vi "SetROI_v4.vi"() -> ()   [LabVIEW 2015]
uses:
  <vilib>/Utility/miscctls.llb/LVPoint32TypeDef.ctl
panel:
  in  "imageselect":u16(ring)
  in  "Add":bool
  in  "Rotate":bool
  in  "Array":T1[](array[typedef])
  in  "no draw":bool
  in  "Scanning Mode":u16(ring) items=["Raster", "Spiral", "resonant"]
  in  "reset angle":bool
  out "Angle":dbl
  in  "Drawing Mode":u16(ring) items=["Image", "Fill Rectangle", "Fill Circle", "Draw Freeform", "Fill Freeform", "Ellipse ", "Line"]
  in  "square matrix":bool
  in  "square pixels":bool
  in  "Ypixels":i32
  in  "Xpixels":i32
  out "Vy-max":dbl
  out "Vx-max":dbl
  out "Vy-min":dbl
  out "Vx-min":dbl
  in  "Cancel Button":bool
  in  "OK Button":bool
  in  "Colormap":u16(ring) items=["Grey", "Red", "Green", "Blue", "Hot", "Winter", "Jet"]
  out "Image":sgl[][](graph)
  # "Note: not idiot proof. if you selected \"image\" as drawing mode, please\nactually scan the image. parameters in the program will be updated to reflect this, \nat the moment there is no flag for whether a selected ROI images has actually been recorded.\nthis will affect accuracy of other drawn ROIs."
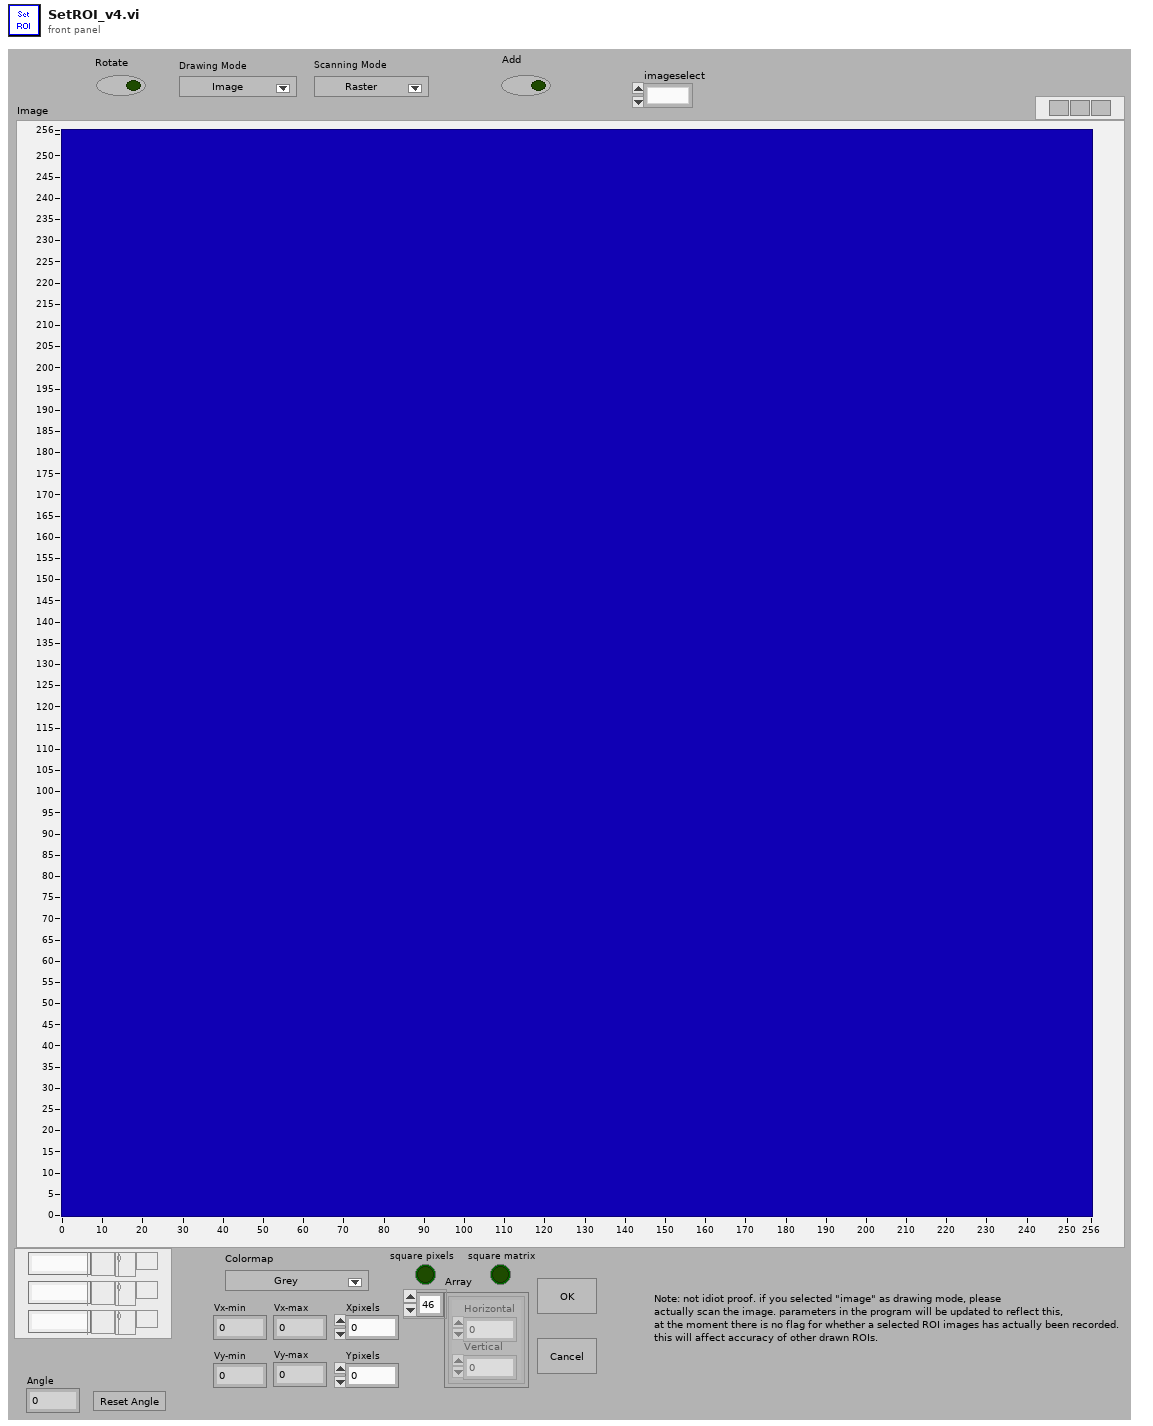
[diagram p1: front panel]
types:
  T1 = typedef "LVPoint32TypeDef.ctl" = cluster{"Horizontal":i32, "Vertical":i32}
  T2 = enum8{"Enabled", "Disabled", "Disabled and Grayed Out"}
  T3 = cluster{"Width":i16, "Style":enum32{"Solid", "Dash", "Dot", "DashDot", "DashDotDot"}}
  T4 = cluster{"StageS":i32, "StageL":i32, "currmeas data dir":path, "image OD":u16, "contour OD":u16, "point OD":u16, "AOlines":tag[], "AIlines":tag[], "CI lines":tag[], "DO lines":tag[], "AO names":string[], "CI names":string[], "AI names":string[], "DO names":string[], "CIextensions":string[], "AIextensions":string[], "Voltage to Ygalvo":i32, "Voltage to Xgalvo":i32, "Voltage to patch":i32, "640 shutter":i32, "2P shutter":i32, "LT timestamp":u32, "Vp":i32, "Ip":i32, "camera trigger":i32, "master data dir":path, "voltage to Zpos":i32, "Vto2P":i32, "640 AO":i32, "488 AO":i32, "532 AO":i32, "640TTL":u32, "488TTL":u32, "532TTL":u32, "Device 1 sampleclock out":tag, "Device 1 Starttrigger out":tag, "Device 2 sampleclock in":tag, "Device 2 StartTrigger in ":tag, "2PODTTL":u32, "488 shutter":u32, "LCVR":u32}
  T5 = typedef "LVRectTypeDef.ctl" = cluster{"Left":i16, "Top":i16, "Right":i16, "Bottom":i16}
  T6 = cluster{"Xpixels":i32, "Vxminref":dbl, "Vxmaxref":dbl, "P":dbl, "Ypixels":i32, "Vyminref":dbl, "Vymaxref":dbl, "srate":sgl, "sAOxy":i32, "timeout":dbl, "type":string, "date":string, "time":string, "Colormap":u16, "Drawing Mode":u16, "Scanning Mode":u16, "square pixels":bool, "square matrix":bool, "Xpixels Img":i32, "Vx-min Img":dbl, "VX-max Img":dbl, "Ypixels Img":i32, "Vy-min Img":dbl, "Vy-max Img ":dbl, "Angle Img":dbl, "autoshutter":bool, "finite":bool, "cont":bool, "wavdet":bool, "measpoints":i32, "avpp":i32, "bufferAO":i32, "bufferAI":i32, "starttick":u32, "waveform":path, "Vx-ref":dbl, "Vy-ref":dbl, "refreshrate":dbl, "refreshbuffer":i32, "tt_cycles":i32, "motorref":refnum<k7>, "mirrorswitch":refnum<k7>, "sample mode":i32, "maxbufferAI":i32, "srateAODO":sgl, "bin":sgl, "Pel":sgl, "Angle draw":dbl, "srate Img":sgl, "ROIimg_plotbounds":T5, "auto OD":bool, "ODfilt":u16, "aAI":i32[], "aCI":i32[], "aAO":u32[], "aDO":u32[], "refwfsize":dbl, "Lifetime":bool, "Vz-Img":dbl, "Vz-ref":dbl, "Vz-reset":dbl, "AIoverride":bool}
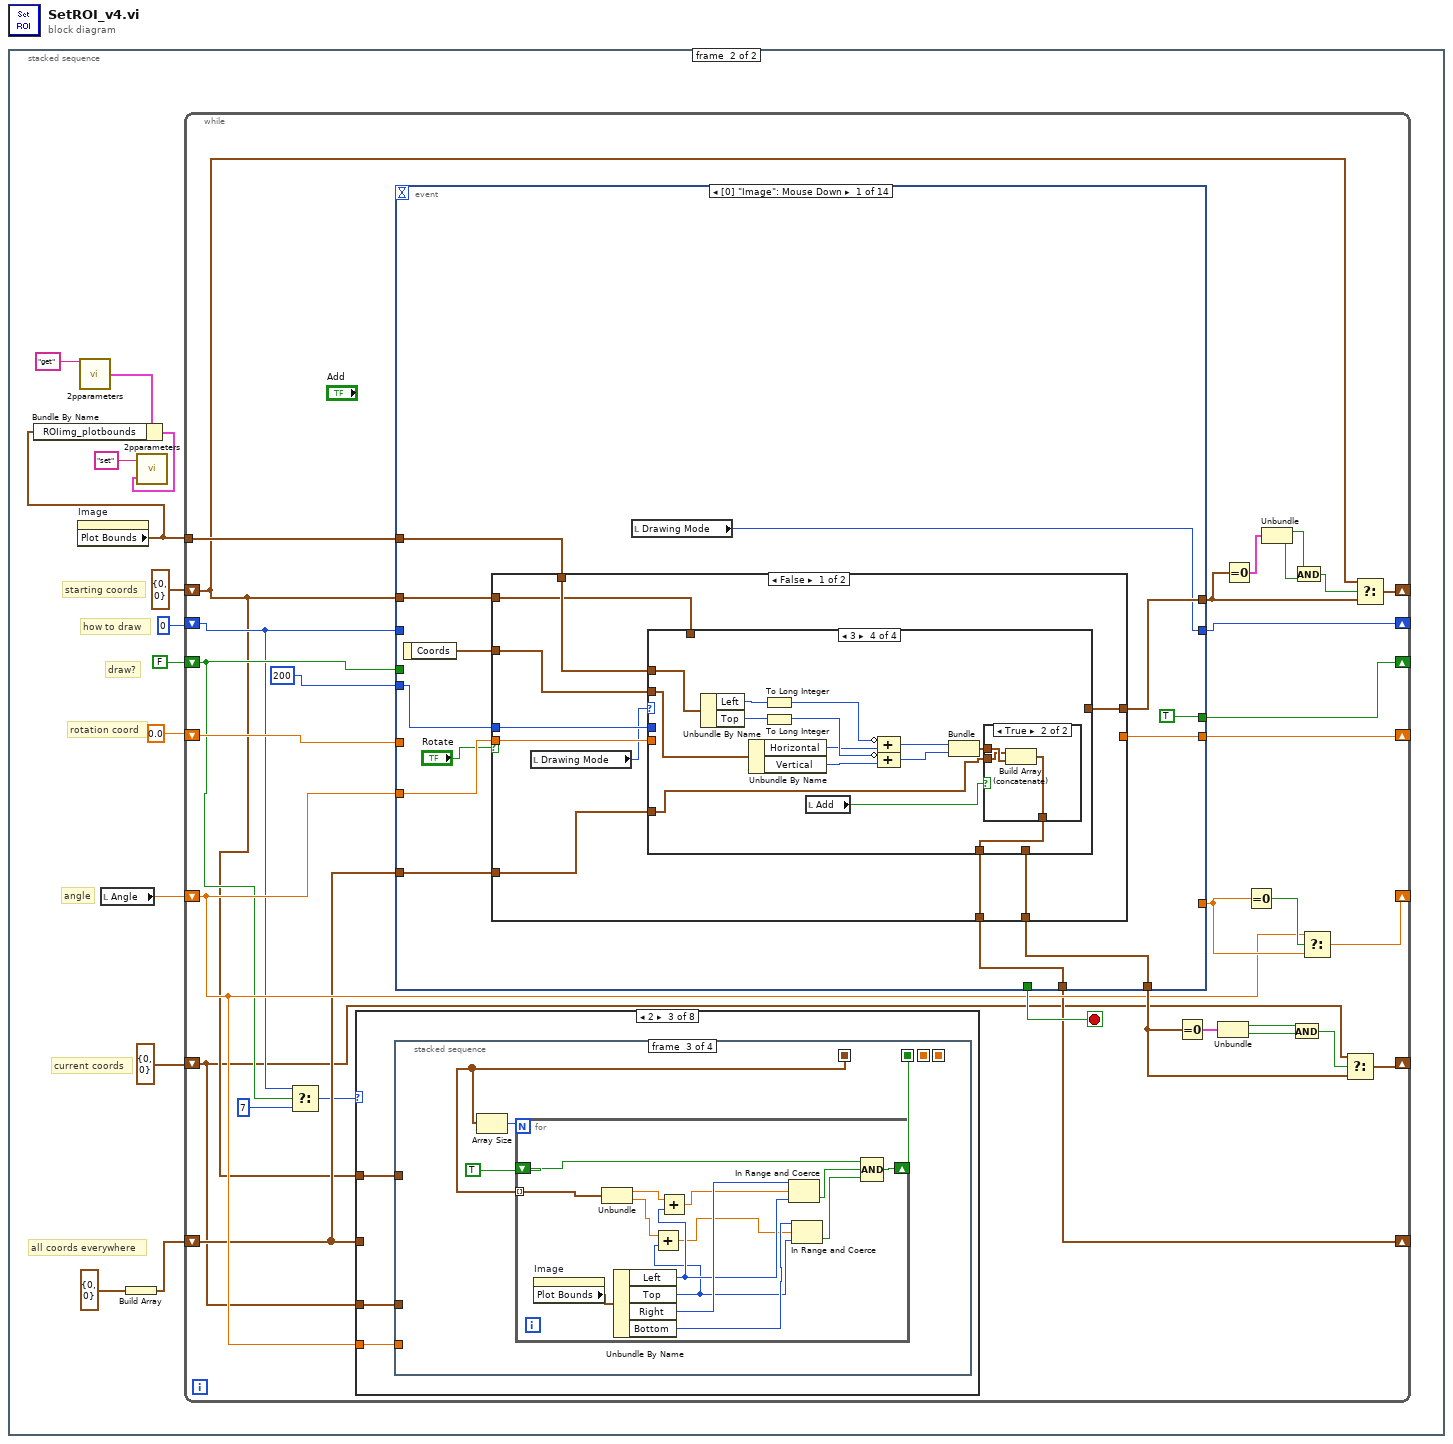
[diagram p0: block diagram]
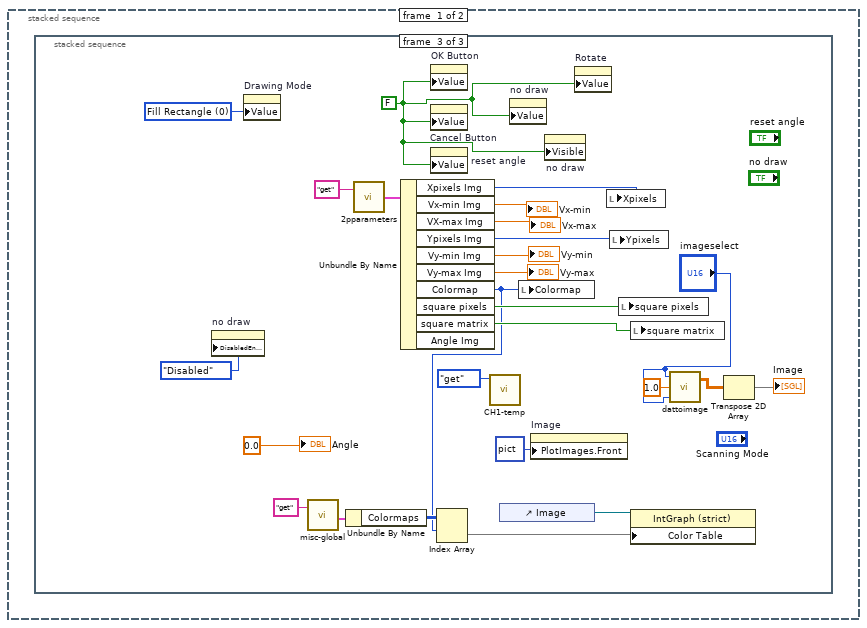
[diagram p2: hidden frame]
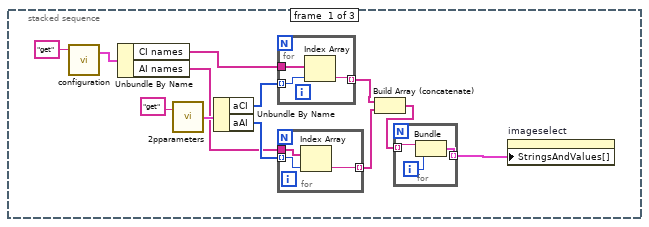
[diagram p3: hidden frame]
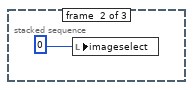
[diagram p4: hidden frame]
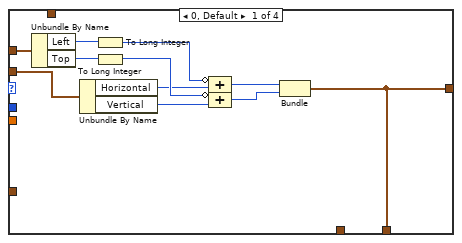
[diagram p5: hidden frame]
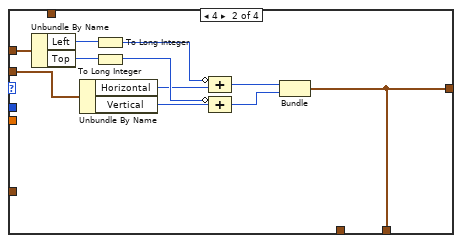
[diagram p6: hidden frame]
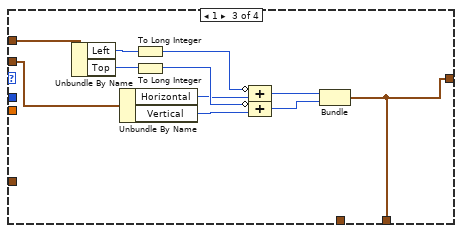
[diagram p7: hidden frame]
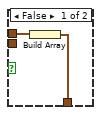
[diagram p8: hidden frame]
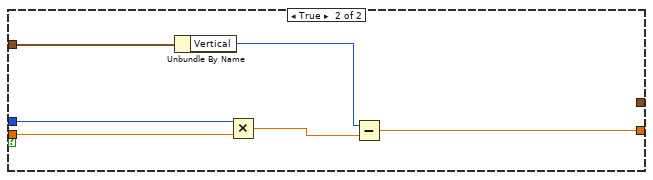
[diagram p9: hidden frame]
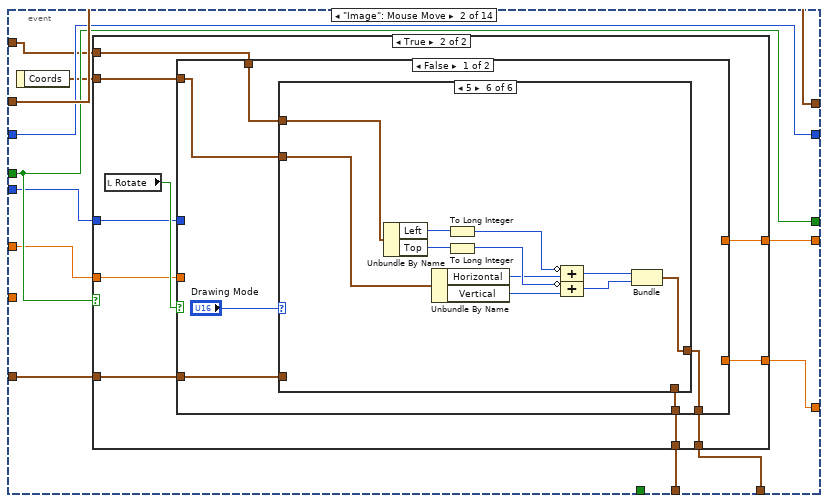
[diagram p10: hidden frame]
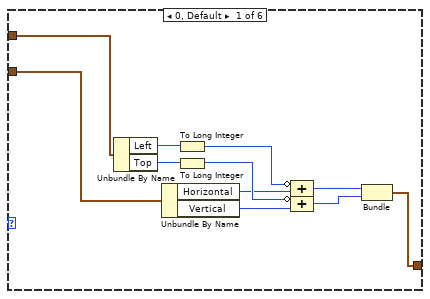
[diagram p12: hidden frame]
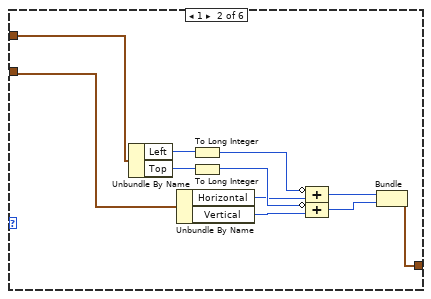
[diagram p13: hidden frame]
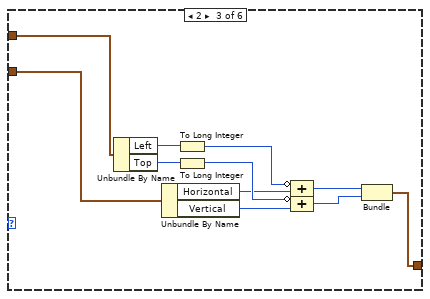
[diagram p14: hidden frame]
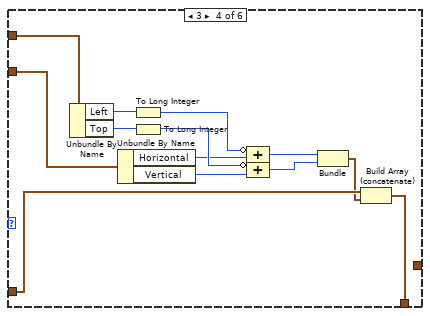
[diagram p15: hidden frame]
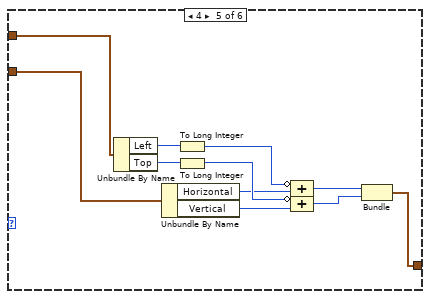
[diagram p16: hidden frame]
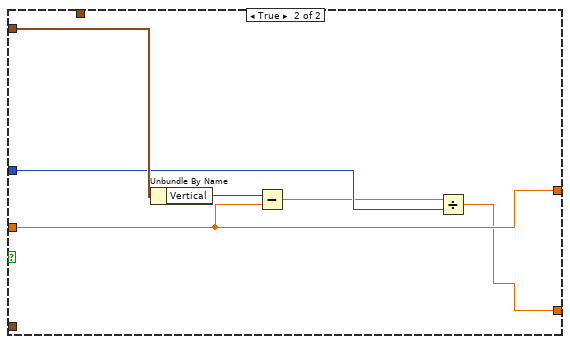
[diagram p17: hidden frame]
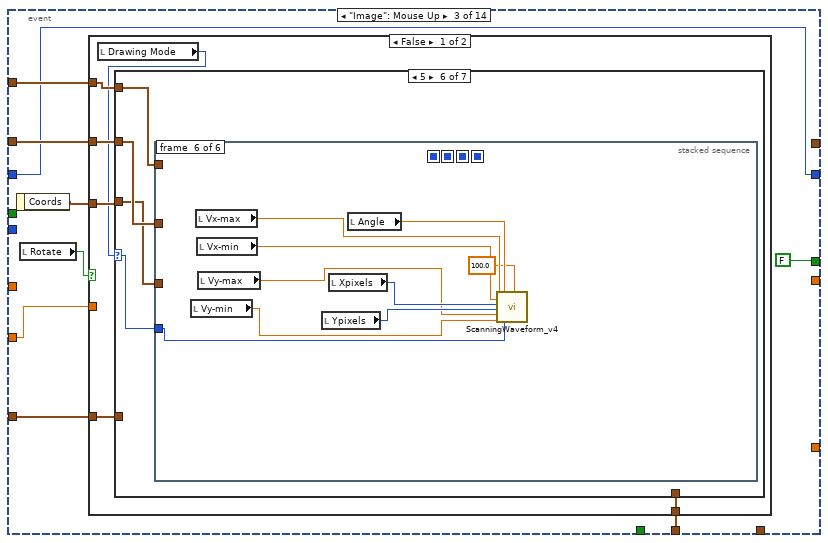
[diagram p18: hidden frame]
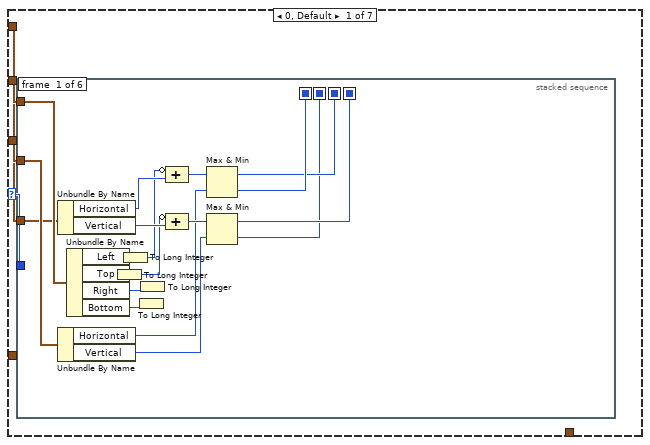
[diagram p19: hidden frame]
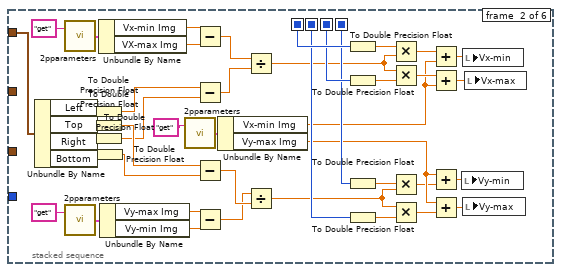
[diagram p20: hidden frame]
diagram:
  n1 = stacked-sequence {
    frame #0 {
      n2 = stacked-sequence {
        frame #0 {
          n3 = call "configuration.vi"("command"="get") -> ("config out"=w5:T4)  [unwired: 2 in, 1 out]
          n4 = Unbundle By Name(w5) -> ("CI names"=w4:string[], "AI names"=w3:string[])
          n5 = call "2pparameters.vi"("command"="get") -> ("params out"=w9:T6)  [unwired: 1 in]
          n6 = Unbundle By Name(w9) -> ("aCI"=w8:i32[], "aAI"=w7:i32[])
          n7 = for {
            tunnel: w8 -> [w20] mode=indexing
            tunnel: w4 -> [w21]
            tunnel: [w19] -> w2 mode=indexing
            n8 = Index Array(array=w21, index=w20) -> (element=w19:string)
          }
          n9 = for {
            tunnel: w7 -> [w17] mode=indexing
            tunnel: w3 -> [w18]
            tunnel: [w16] -> w1 mode=indexing
            n10 = Index Array(array=w18, index=w17) -> (element=w16:string)
          }
          n11 = Build Array (concatenate)(w2, w1) -> (w11:string[])
          n12 = for {
            tunnel: w11 -> [w14] mode=indexing
            tunnel: [w13] -> w12 mode=indexing
            i -> [w15]
            n13 = Bundle("String"=w14, w15) -> (w13:cluster{"String":string, i32})  [unwired: 1 in]
          }
          n14 = property on="imageselect" class="Ring (strict)"("StringsAndValues[]"=w12) -> ()  [unwired: 2 in, 2 out]
        }
        frame #1 {
          n15 = local write "imageselect"(0) -> ()
        }
        frame #2 {
          w34 = u16 0 items=["Fill Rectangle", "Fill Circle", "Draw Freeform", "Fill Freeform"] ("Drawing Mode")
          w33 = FALSE ("Cancel Button")
          n16 = property on="no draw" class="Bool (strict)"("DisabledEnum"=T2."Disabled" ("Disabled")) -> ()  [unwired: 2 in, 2 out]
          n17 = property on="Drawing Mode" class="Ring (strict)"("Value"=w34) -> ()  [unwired: 2 in, 2 out]
          n18 = call "misc-global.vi"("command"="get") -> ("misc out"=w29:cluster{"Colormaps":u32[][]})  [unwired: 1 in]
          n19 = Unbundle By Name(w29) -> ("Colormaps"=w28:u32[][])
          n20 = call "2pparameters.vi"("command"="get") -> ("params out"=w47:T6)  [unwired: 1 in]
          n21 = Unbundle By Name(w47) -> ("Xpixels Img"=w40:i32, "Vx-min Img"=→"Vx-min":dbl, "VX-max Img"=→"Vx-max":dbl, "Ypixels Img"=w39:i32, "Vy-min Img"=→"Vy-min":dbl, "Vy-max Img"=→"Vy-max":dbl, "Colormap"=w26:u16, "square pixels"=w41:bool, "square matrix"=w42:bool)  [unwired: 1 out]
          n22 = property on="OK Button" class="Bool (strict)"("Value"=w33) -> ()  [unwired: 2 in, 2 out]
          n23 = property on="Cancel Button" class="Bool (strict)"("Value"=w33) -> ()  [unwired: 2 in, 2 out]
          n24 = property on="reset angle" class="Bool (strict)"("Value"=w33) -> ()  [unwired: 2 in, 2 out]
          n25 = Index Array(array=w28, index (row)=w26) -> (element=w27:u32[])  [unwired: 1 in]
          n26 = call "CH1-temp.vi"("command"=enum16{"get", "set", "clear", "add row"}."get") -> ()  [unwired: 3 in, 2 out]
          n27 = control-ref of="Image"() -> (w31:refnum<vi>)
          n28 = property on="no draw" class="Bool (strict)"("Value"=w33) -> ()  [unwired: 2 in, 2 out]
          n29 = local write "Colormap"(w26) -> ()
          n30 = property on="Image" class="IntGraph (strict)"("PlotImages.Front"=picture data[5B] ("Plot Images:Front")) -> ()  [unwired: 2 in, 2 out]
          n31 = property on="no draw" class="Bool (strict)"("Visible"=w33) -> ()  [unwired: 2 in, 2 out]
          n32 = property on="Rotate" class="Bool (strict)"("Value"=w33) -> ()  [unwired: 2 in, 2 out]
          n33 = local write "Xpixels"(w40) -> ()
          n34 = local write "Ypixels"(w39) -> ()
          n35 = local write "square pixels"(w41) -> ()
          n36 = local write "square matrix"(w42) -> ()
          n37 = property class="IntGraph (strict)"(reference=w31, "Color Table"=w27) -> ()  [unwired: 1 in, 2 out]
          n38 = call "dattoimage.vi"("image2list"="imageselect", "Current Average"=sgl 1.0, "image1list"="imageselect") -> ("image 1 array out"=w24:sgl[][])  [unwired: 1 out]
          n39 = Transpose 2D Array(2D array=w24) -> (transposed array=→"Image":sgl[][])
          "Angle" <- 0.0
        }
      }
    }
    frame #1 {
      # "draw?"
      # "all coords everywhere"
      # "current coords"
      # "angle"
      # "rotation coord"
      # "how to draw"
      # "starting coords"
      n40 = property on="Image" class="IntGraph (strict)"() -> ("Plot Bounds"=w50:T5)  [unwired: 2 in, 2 out]
      n41 = call "2pparameters.vi"("command"="get") -> ("params out"=w51:T6)  [unwired: 1 in]
      n42 = Bundle By Name(cluster=w51, "ROIimg_plotbounds"=w50) -> (w49:T6)
      n43 = local read "Angle"() -> (w56:dbl)
      n44 = Build Array(T1 {"Horizontal"=0, "Vertical"=0} ("Coords")) -> (w57:T1[])
      n45 = call "2pparameters.vi"("Params in"=w49, "command"="set") -> ()  [unwired: 1 out]
      n46 = while {
        shift-right: [w85] -> _
        shift-left: T1 {"Horizontal"=0, "Vertical"=0} ("Coords") -> [w64]
        shift-right: [w62] -> _
        shift-left: 0 -> [w65]
        tunnel: w50 -> [w91]
        shift-right: [w82] -> _
        shift-left: w56 -> [w72]
        shift-right: [w80] -> _
        shift-left: T1 {"Horizontal"=0, "Vertical"=0} ("Coords") -> [w63]
        shift-right: [w75] -> _
        shift-left: 0.0 -> [w73]
        shift-right: [w70] -> _
        shift-left: w57 -> [w71]
        shift-right: [w67] -> _
        shift-left: FALSE -> [w66]
        stop <- w92 stop-if-true
        n47 = Select(t=w65, s=w66, f=7) -> (s? t:f=w68:i32)
        n48 = case shown="2" w68 {
          tunnel: w63 -> [w1505 w1559 w1613 _ _ w1678 _ _]
          tunnel: w64 -> [w1506 w1560 w1614 _ _ w1679 w1728 _]
          tunnel: w72 -> [w1504 w1558 w1612 _ _ w1677 _ _]
          tunnel: w71 -> [_ _ _ w1665 w1672 _ _ _]
          frame 0, Default {
            n49 = stacked-sequence {
              seq-local: [w1507 _ _] -> [_ w1531 w1550]
              seq-local: [_ w1532 _] -> [_ _ w1549]
              tunnel: w1506 -> [w1530 _ _]
              tunnel: w1505 -> [w1511 _ _]
              tunnel: w1504 -> [w1510 _ _]
              frame #0 {
                n50 = Unbundle By Name(w1530) -> ("Horizontal"=w1508:i32, "Vertical"=w1509:i32)
                n51 = Unbundle By Name(w1511) -> ("Horizontal"=w1514:i32, "Vertical"=w1515:i32)
                n52 = Add(x=w1508, y=w1514) -> (x+y=w1519:i32)
                n53 = Subtract(x=w1508, y=w1514) -> (x-y=w1518:i32)
                n54 = Subtract(x=w1509, y=w1515) -> (x-y=w1516:i32)
                n55 = Add(x=w1509, y=w1515) -> (x+y=w1517:i32)
                n56 = formula code="p1x = xc/2+xs/2*cos(t)-ys/2*sin(t);\np1y = yc/2+xs/2*sin(t)+ys/2*cos(t);\np2x = xc/2+xs/2*cos(t)+ys/2*sin(t);\np2y = yc/2+xs/2*sin(t)-ys/2*cos(t);\np3x = xc/2-xs/2*cos(t)+ys/2*sin(t);\np3y = yc/2-xs/2*sin(t)-ys/2*cos(t);\np4x = xc/2-xs/2*cos(t)-ys/2*sin(t);\np4y = yc/2-xs/2*sin(t)+ys/2*cos(t);"("xc"=w1519, "xs"=w1518, "yc"=w1517, "ys"=w1516, "t"=w1510) -> ("p2x"=w1524:dbl, "p1x"=w1520:dbl, "p3x"=w1526:dbl, "p4x"=w1528:dbl, "p1y"=w1521:dbl, "p2y"=w1525:dbl, "p3y"=w1527:dbl, "p4y"=w1529:dbl)
                n57 = Bundle("p2x"=w1524, "p2y"=w1525) -> (w1513:cluster{"p2x":dbl, "p2y":dbl})  [unwired: 1 out]
                n58 = Bundle("p1x"=w1520, "p1y"=w1521) -> (w1512:cluster{"p1x":dbl, "p1y":dbl})  [unwired: 1 out]
                n59 = Bundle("p4x"=w1528, "p4y"=w1529) -> (w1523:cluster{"p4x":dbl, "p4y":dbl})  [unwired: 1 out]
                n60 = Bundle("p3x"=w1526, "p3y"=w1527) -> (w1522:cluster{"p3x":dbl, "p3y":dbl})  [unwired: 1 out]
                n61 = Build Array(w1512, w1513, w1522, w1523, w1512) -> (w1507:cluster{"p1x":dbl, "p1y":dbl}[])
              }
              frame #1 {
                n62 = Array Size(array=w1531) -> (size(s)=w1534:i32)
                n63 = for {
                  N: w1534 -> [_]
                  shift-right: [w1547] -> w1532
                  shift-left: TRUE -> [w1545]
                  tunnel: w1531 -> [w1548] mode=indexing
                  n64 = property on="Image" class="IntGraph (strict)"() -> ("Plot Bounds"=w1543:T5)  [unwired: 2 in, 2 out]
                  n65 = Unbundle By Name(w1548) -> ("p1x"=w1540:dbl, "p1y"=w1536:dbl)
                  n66 = Unbundle By Name(w1543) -> ("Left"=w1541:i16, "Top"=w1537:i16, "Right"=w1542:i16, "Bottom"=w1538:i16)
                  n67 = Add(x=w1536, y=w1537) -> (x+y=w1535:dbl)
                  n68 = Add(x=w1540, y=w1541) -> (x+y=w1539:dbl)
                  n69 = In Range and Coerce(upper limit=w1542, x=w1539, lower limit=w1541) -> (In Range?=w1546:bool)  [unwired: 1 out]
                  n70 = In Range and Coerce(upper limit=w1538, x=w1535, lower limit=w1537) -> (In Range?=w1544:bool)  [unwired: 1 out]
                  n71 = Compound Arithmetic op=AND(w1545, w1546, w1544) -> (w1547:bool)
                }
              }
              frame #2 {
                n72 = case shown="True" w1549 {
                  tunnel: w1550 -> [_ w1554]
                  frame False {
                    n73 = property on="no draw" class="Bool (strict)"("DisabledEnum"=T2."Enabled" ("Disabled")) -> ()  [unwired: 2 in, 2 out]
                    n74 = property on="no draw" class="Bool (strict)"("Visible"=TRUE) -> ()  [unwired: 2 in, 2 out]
                    n75 = property on="OK Button" class="Bool (strict)"("DisabledEnum"=T2."Disabled" ("Disabled")) -> ()  [unwired: 2 in, 2 out]
                  }
                  frame True {
                    n76 = call <vilib>:"Draw Multiple Lines.vi"("line endpoints"=w1554, "color(black)"=u32 16774656, "pen"=T3 {"Width"=3, "Style"=enum."Dash"}) -> ("new picture"=w1556:picture)  [unwired: 6 in]
                    n77 = property on="Image" class="IntGraph (strict)"("PlotImages.Front"=w1556) -> ()  [unwired: 2 in, 2 out]
                  }
                }
              }
            }
          }
          frame 1 {
            n78 = stacked-sequence {
              seq-local: [w1561 _ _] -> [_ w1585 w1604]
              seq-local: [_ w1586 _] -> [_ _ w1603]
              tunnel: w1560 -> [w1584 _ _]
              tunnel: w1559 -> [w1565 _ _]
              tunnel: w1558 -> [w1564 _ _]
              frame #0 {
                n79 = Unbundle By Name(w1584) -> ("Horizontal"=w1562:i32, "Vertical"=w1563:i32)
                n80 = Unbundle By Name(w1565) -> ("Horizontal"=w1568:i32, "Vertical"=w1569:i32)
                n81 = Add(x=w1562, y=w1568) -> (x+y=w1573:i32)
                n82 = Subtract(x=w1562, y=w1568) -> (x-y=w1572:i32)
                n83 = Subtract(x=w1563, y=w1569) -> (x-y=w1570:i32)
                n84 = Add(x=w1563, y=w1569) -> (x+y=w1571:i32)
                n85 = formula code="p1x = xc/2+xs/2*cos(t)-ys/2*sin(t);\np1y = yc/2+xs/2*sin(t)+ys/2*cos(t);\np2x = xc/2+xs/2*cos(t)+ys/2*sin(t);\np2y = yc/2+xs/2*sin(t)-ys/2*cos(t);\np3x = xc/2-xs/2*cos(t)+ys/2*sin(t);\np3y = yc/2-xs/2*sin(t)-ys/2*cos(t);\np4x = xc/2-xs/2*cos(t)-ys/2*sin(t);\np4y = yc/2-xs/2*sin(t)+ys/2*cos(t);"("xc"=w1573, "xs"=w1572, "yc"=w1571, "ys"=w1570, "t"=w1564) -> ("p2x"=w1578:dbl, "p1x"=w1574:dbl, "p3x"=w1580:dbl, "p4x"=w1582:dbl, "p1y"=w1575:dbl, "p2y"=w1579:dbl, "p3y"=w1581:dbl, "p4y"=w1583:dbl)
                n86 = Bundle("p2x"=w1578, "p2y"=w1579) -> (w1567:cluster{"p2x":dbl, "p2y":dbl})  [unwired: 1 out]
                n87 = Bundle("p1x"=w1574, "p1y"=w1575) -> (w1566:cluster{"p1x":dbl, "p1y":dbl})  [unwired: 1 out]
                n88 = Bundle("p4x"=w1582, "p4y"=w1583) -> (w1577:cluster{"p4x":dbl, "p4y":dbl})  [unwired: 1 out]
                n89 = Bundle("p3x"=w1580, "p3y"=w1581) -> (w1576:cluster{"p3x":dbl, "p3y":dbl})  [unwired: 1 out]
                n90 = Build Array(w1566, w1567, w1576, w1577, w1566) -> (w1561:cluster{"p1x":dbl, "p1y":dbl}[])
              }
              frame #1 {
                n91 = Array Size(array=w1585) -> (size(s)=w1588:i32)
                n92 = for {
                  N: w1588 -> [_]
                  shift-right: [w1601] -> w1586
                  shift-left: TRUE -> [w1599]
                  tunnel: w1585 -> [w1602] mode=indexing
                  n93 = property on="Image" class="IntGraph (strict)"() -> ("Plot Bounds"=w1597:T5)  [unwired: 2 in, 2 out]
                  n94 = Unbundle By Name(w1602) -> ("p1x"=w1594:dbl, "p1y"=w1590:dbl)
                  n95 = Unbundle By Name(w1597) -> ("Left"=w1595:i16, "Top"=w1591:i16, "Right"=w1596:i16, "Bottom"=w1592:i16)
                  n96 = Add(x=w1590, y=w1591) -> (x+y=w1589:dbl)
                  n97 = Add(x=w1594, y=w1595) -> (x+y=w1593:dbl)
                  n98 = In Range and Coerce(upper limit=w1596, x=w1593, lower limit=w1595) -> (In Range?=w1600:bool)  [unwired: 1 out]
                  n99 = In Range and Coerce(upper limit=w1592, x=w1589, lower limit=w1591) -> (In Range?=w1598:bool)  [unwired: 1 out]
                  n100 = Compound Arithmetic op=AND(w1599, w1600, w1598) -> (w1601:bool)
                }
              }
              frame #2 {
                n101 = case shown="True" w1603 {
                  tunnel: w1604 -> [_ w1608]
                  frame False {
                    n102 = property on="no draw" class="Bool (strict)"("DisabledEnum"=T2."Enabled" ("Disabled")) -> ()  [unwired: 2 in, 2 out]
                    n103 = property on="no draw" class="Bool (strict)"("Visible"=TRUE) -> ()  [unwired: 2 in, 2 out]
                    n104 = property on="OK Button" class="Bool (strict)"("DisabledEnum"=T2."Disabled" ("Disabled")) -> ()  [unwired: 2 in, 2 out]
                  }
                  frame True {
                    n105 = call <vilib>:"Draw Multiple Lines.vi"("line endpoints"=w1608, "color(black)"=u32 16774656, "pen"=T3 {"Width"=3, "Style"=enum."Dash"}) -> ("new picture"=w1610:picture)  [unwired: 6 in]
                    n106 = property on="Image" class="IntGraph (strict)"("PlotImages.Front"=w1610) -> ()  [unwired: 2 in, 2 out]
                  }
                }
              }
            }
          }
          frame 2 {
            n107 = stacked-sequence {
              seq-local: [_ w1628 _ _] -> [_ _ w1637 w1655]
              seq-local: [_ _ w1636 _] -> [_ _ _ w1654]
              seq-local: [w1618 _ _ _] -> [_ w1629 _ _]
              seq-local: [w1617 _ _ _] -> [_ w1627 _ _]
              tunnel: w1614 -> [w1625 _ _ _]
              tunnel: w1613 -> [w1622 _ _ _]
              tunnel: w1612 -> [w1619 _ _ _]
              frame #0 {
                n108 = Unbundle By Name(w1625) -> ("Horizontal"=w1616:i32, "Vertical"=w1615:i32)
                n109 = Unbundle By Name(w1622) -> ("Horizontal"=w1623:i32, "Vertical"=w1624:i32)
                n110 = Subtract(x=w1616, y=w1623) -> (x-y=w1621:i32)
                n111 = Subtract(x=w1615, y=w1624) -> (x-y=w1620:i32)
                n112 = script code="t=2*pi*(0:0.01:1);\nX=A.*cos(t).*cos(phi)-B.*sin(t).*sin(phi)+Xc\nY=A.*cos(t).*sin(phi)+B.*sin(t).*cos(phi)+Yc"("Xc"=w1616, "Yc"=w1615, "A"=w1621, "B"=w1620, "phi"=w1619) -> ("X"=w1618:dbl[], "Y"=w1617:dbl[])  [unwired: 1 in, 1 out]
              }
              frame #1 {
                n113 = Array Size(array=w1627) -> (size(s)=w1630:i32)
                n114 = for {
                  N: w1630 -> [_]
                  tunnel: w1629 -> [w1635] mode=indexing
                  tunnel: w1627 -> [w1634] mode=indexing
                  shift-right: [w1631] -> w1628
                  shift-left: cluster{dbl, dbl}[] [] -> [w1632]
                  n115 = Bundle(w1635, w1634) -> (w1633:cluster{dbl, dbl})  [unwired: 1 out]
                  n116 = Build Array (concatenate)(w1632, w1633) -> (w1631:cluster{dbl, dbl}[])
                }
              }
              frame #2 {
                n117 = Array Size(array=w1637) -> (size(s)=w1639:i32)
                n118 = for {
                  N: w1639 -> [_]
                  shift-right: [w1652] -> w1636
                  shift-left: TRUE -> [w1650]
                  tunnel: w1637 -> [w1653] mode=indexing
                  n119 = property on="Image" class="IntGraph (strict)"() -> ("Plot Bounds"=w1648:T5)  [unwired: 2 in, 2 out]
                  n120 = Unbundle(w1653) -> (w1645:dbl, w1641:dbl)
                  n121 = Unbundle By Name(w1648) -> ("Left"=w1646:i16, "Top"=w1642:i16, "Right"=w1647:i16, "Bottom"=w1643:i16)
                  n122 = Add(x=w1641, y=w1642) -> (x+y=w1640:dbl)
                  n123 = Add(x=w1645, y=w1646) -> (x+y=w1644:dbl)
                  n124 = In Range and Coerce(upper limit=w1647, x=w1644, lower limit=w1646) -> (In Range?=w1651:bool)  [unwired: 1 out]
                  n125 = In Range and Coerce(upper limit=w1643, x=w1640, lower limit=w1642) -> (In Range?=w1649:bool)  [unwired: 1 out]
                  n126 = Compound Arithmetic op=AND(w1650, w1651, w1649) -> (w1652:bool)
                }
              }
              frame #3 {
                n127 = case shown="True" w1654 {
                  tunnel: w1655 -> [_ w1659]
                  frame False {
                    n128 = property on="no draw" class="Bool (strict)"("DisabledEnum"=T2."Enabled" ("Disabled")) -> ()  [unwired: 2 in, 2 out]
                    n129 = property on="no draw" class="Bool (strict)"("Visible"=TRUE) -> ()  [unwired: 2 in, 2 out]
                    n130 = property on="OK Button" class="Bool (strict)"("DisabledEnum"=T2."Disabled" ("Disabled")) -> ()  [unwired: 2 in, 2 out]
                  }
                  frame True {
                    n131 = call <vilib>:"Draw Multiple Lines.vi"("line endpoints"=w1659, "color(black)"=u32 16774656, "pen"=T3 {"Width"=3, "Style"=enum."Dash"}) -> ("new picture"=w1661:picture)  [unwired: 6 in]
                    n132 = property on="Image" class="IntGraph (strict)"("PlotImages.Front"=w1661) -> ()  [unwired: 2 in, 2 out]
                  }
                }
              }
            }
          }
          frame 3 {
            n133 = Index Array(array=w1665, index=0) -> (element=w1666:T1)
            n134 = Build Array (concatenate)(w1665, w1666) -> (w1663:T1[])
            n135 = call <vilib>:"Draw Multiple Lines.vi"("line endpoints"=w1663, "color(black)"=u32 16774656, "pen"=T3 {"Width"=3, "Style"=enum."Dot"}) -> ("new picture"=w1668:picture)  [unwired: 6 in]
            n136 = property on="Image" class="IntGraph (strict)"("PlotImages.Front"=w1668) -> ()  [unwired: 2 in, 2 out]
          }
          frame 4 {
            n137 = Index Array(array=w1672, index=0) -> (element=w1673:T1)
            n138 = Build Array (concatenate)(w1672, w1673) -> (w1670:T1[])
            n139 = call <vilib>:"Draw Multiple Lines.vi"("line endpoints"=w1670, "color(black)"=u32 16774656, "pen"=T3 {"Width"=3, "Style"=enum."Solid"}) -> ("new picture"=w1675:picture)  [unwired: 6 in]
            n140 = property on="Image" class="IntGraph (strict)"("PlotImages.Front"=w1675) -> ()  [unwired: 2 in, 2 out]
          }
          frame 5 {
            n141 = stacked-sequence {
              seq-local: [_ w1693 _ _] -> [_ _ w1702 w1720]
              seq-local: [_ _ w1701 _] -> [_ _ _ w1719]
              seq-local: [w1683 _ _ _] -> [_ w1694 _ _]
              seq-local: [w1682 _ _ _] -> [_ w1692 _ _]
              tunnel: w1679 -> [w1690 _ _ _]
              tunnel: w1678 -> [w1687 _ _ _]
              tunnel: w1677 -> [w1684 _ _ _]
              frame #0 {
                n142 = Unbundle By Name(w1690) -> ("Horizontal"=w1681:i32, "Vertical"=w1680:i32)
                n143 = Unbundle By Name(w1687) -> ("Horizontal"=w1688:i32, "Vertical"=w1689:i32)
                n144 = Subtract(x=w1681, y=w1688) -> (x-y=w1686:i32)
                n145 = Subtract(x=w1680, y=w1689) -> (x-y=w1685:i32)
                n146 = script code="t=2*pi*(0:0.01:1);\nX=A.*cos(t).*cos(phi)-B.*sin(t).*sin(phi)+Xc\nY=A.*cos(t).*sin(phi)+B.*sin(t).*cos(phi)+Yc"("Xc"=w1681, "Yc"=w1680, "A"=w1686, "B"=w1685, "phi"=w1684) -> ("X"=w1683:dbl[], "Y"=w1682:dbl[])  [unwired: 1 in, 1 out]
              }
              frame #1 {
                n147 = Array Size(array=w1692) -> (size(s)=w1695:i32)
                n148 = for {
                  N: w1695 -> [_]
                  tunnel: w1694 -> [w1700] mode=indexing
                  tunnel: w1692 -> [w1699] mode=indexing
                  shift-right: [w1696] -> w1693
                  shift-left: cluster{dbl, dbl}[] [] -> [w1697]
                  n149 = Bundle(w1700, w1699) -> (w1698:cluster{dbl, dbl})  [unwired: 1 out]
                  n150 = Build Array (concatenate)(w1697, w1698) -> (w1696:cluster{dbl, dbl}[])
                }
              }
              frame #2 {
                n151 = Array Size(array=w1702) -> (size(s)=w1704:i32)
                n152 = for {
                  N: w1704 -> [_]
                  shift-right: [w1717] -> w1701
                  shift-left: TRUE -> [w1715]
                  tunnel: w1702 -> [w1718] mode=indexing
                  n153 = property on="Image" class="IntGraph (strict)"() -> ("Plot Bounds"=w1713:T5)  [unwired: 2 in, 2 out]
                  n154 = Unbundle(w1718) -> (w1710:dbl, w1706:dbl)
                  n155 = Unbundle By Name(w1713) -> ("Left"=w1711:i16, "Top"=w1707:i16, "Right"=w1712:i16, "Bottom"=w1708:i16)
                  n156 = Add(x=w1706, y=w1707) -> (x+y=w1705:dbl)
                  n157 = Add(x=w1710, y=w1711) -> (x+y=w1709:dbl)
                  n158 = In Range and Coerce(upper limit=w1712, x=w1709, lower limit=w1711) -> (In Range?=w1716:bool)  [unwired: 1 out]
                  n159 = In Range and Coerce(upper limit=w1708, x=w1705, lower limit=w1707) -> (In Range?=w1714:bool)  [unwired: 1 out]
                  n160 = Compound Arithmetic op=AND(w1715, w1716, w1714) -> (w1717:bool)
                }
              }
              frame #3 {
                n161 = case shown="True" w1719 {
                  tunnel: w1720 -> [_ w1724]
                  frame False {
                    n162 = property on="no draw" class="Bool (strict)"("DisabledEnum"=T2."Enabled" ("Disabled")) -> ()  [unwired: 2 in, 2 out]
                    n163 = property on="no draw" class="Bool (strict)"("Visible"=TRUE) -> ()  [unwired: 2 in, 2 out]
                    n164 = property on="OK Button" class="Bool (strict)"("DisabledEnum"=T2."Disabled" ("Disabled")) -> ()  [unwired: 2 in, 2 out]
                  }
                  frame True {
                    n165 = call <vilib>:"Draw Multiple Lines.vi"("line endpoints"=w1724, "color(black)"=u32 16774656, "pen"=T3 {"Width"=3, "Style"=enum."Dash"}) -> ("new picture"=w1726:picture)  [unwired: 6 in]
                    n166 = property on="Image" class="IntGraph (strict)"("PlotImages.Front"=w1726) -> ()  [unwired: 2 in, 2 out]
                  }
                }
              }
            }
          }
          frame 6 {
            n167 = call <vilib>:"Draw Line.vi"("end point"=w1728, "color(black)"=u32 16774656, "pen"=T3 {"Width"=3, "Style"=enum."Dash"}) -> ("new picture"=w1730:picture)  [unwired: 6 in]
            n168 = property on="Image" class="IntGraph (strict)"("PlotImages.Front"=w1730) -> ()  [unwired: 2 in, 2 out]
          }
          frame 7 {
          }
        }
        n169 = event shown="[0] \"Image\": Mouse Down" {
          selector: _ -> [_ _ _ _ _ _ _ _ _ _ _ _ _ _]
          dyn-events: _ -> [_ _ _ _ _ _ _ _ _ _ _ _ _ _]
          timeout: _ -> [_ _ _ _ _ _ _ _ _ _ _ _ _ _]
          tunnel: [w104 w185 _ _ _ _ _ _ _ _ _ _ _ _] -> w86
          tunnel: w64 -> [w103 w185 w284 _ _ _ _ _ _ _ w1444 _ _ _]
          tunnel: w65 -> [_ w184 w281 _ _ _ _ _ _ _ _ _ _ _]
          tunnel: [w94 w184 w281 _ _ _ _ _ _ 0 _ _ _ _] -> w62
          tunnel: w91 -> [w105 w177 w285 _ _ _ _ _ _ _ _ _ _ _]
          tunnel: [_ _ _ _ _ _ _ _ _ _ _ _ w1451 w1494] -> w92
          tunnel: [_ w178 _ _ _ _ _ _ _ 6.283185307179586 _ _ _ _] -> w83
          tunnel: [w102 w176 _ _ _ _ _ _ _ _ w1444 _ _ _] -> w79
          tunnel: [w101 w179 _ _ _ _ _ _ _ _ _ _ _ _] -> w75
          tunnel: w73 -> [_ w180 _ _ _ _ _ _ _ _ _ _ _ _]
          tunnel: 200 -> [w100 w181 _ _ _ _ _ _ _ _ _ _ _ _]
          tunnel: w72 -> [w99 _ w279 _ _ _ _ _ _ _ _ _ _ _]
          tunnel: [w97 w174 w277 _ _ _ _ _ _ _ _ _ _ _] -> w70
          tunnel: w71 -> [w93 w175 w280 _ _ _ _ _ _ _ _ _ _ _]
          tunnel: [TRUE w183 FALSE _ _ _ _ _ _ _ _ _ _ _] -> w67
          tunnel: w66 -> [_ w183 _ _ _ _ _ _ _ _ _ _ _ _]
          event "Image": Mouse Down {
            n170 = event-data() -> ("Coords"=w98:T1)  [unwired: 1 in]
            n171 = case shown="False" "Rotate" {
              tunnel: w105 -> [w115 _]
              tunnel: [w114 _] -> w104
              tunnel: w103 -> [w113 _]
              tunnel: [w112 _] -> w102
              tunnel: [_ w169] -> w101
              tunnel: w100 -> [w111 w172]
              tunnel: w99 -> [w110 w171]
              tunnel: w98 -> [w109 w168]
              tunnel: [w108 _] -> w97
              tunnel: w93 -> [w106 _]
              frame False {
                n172 = local read "Drawing Mode"() -> (w107:u16)
                n173 = case shown="3" w107 {
                  tunnel: w115 -> [w121 w132 w139 w152]
                  tunnel: [w116 w127 w138 _] -> w114
                  tunnel: w113 -> [_ _ _ _]
                  tunnel: [w116 w127 w138 _] -> w112
                  tunnel: w111 -> [_ _ _ _]
                  tunnel: w110 -> [_ _ _ _]
                  tunnel: w109 -> [w126 w137 w140 w151]
                  tunnel: [_ _ _ w162] -> w108
                  tunnel: w106 -> [_ _ _ w149]
                  frame 0, Default {
                    n174 = Unbundle By Name(w121) -> ("Left"=w125:i16, "Top"=w123:i16)
                    n175 = Unbundle By Name(w126) -> ("Horizontal"=w119:i32, "Vertical"=w120:i32)
                    n176 = To Long Integer(number=w125) -> (32bit integer=w124:i32)
                    n177 = To Long Integer(number=w123) -> (32bit integer=w122:i32)
                    n178 = Compound Arithmetic op=ADD(invert w124, w119) -> (w118:i32)
                    n179 = Compound Arithmetic op=ADD(invert w122, w120) -> (w117:i32)
                    n180 = Bundle(w118, w117) -> (w116:cluster{i32, i32})  [unwired: 1 in]
                  }
                  frame 4 {
                    n181 = Unbundle By Name(w132) -> ("Left"=w136:i16, "Top"=w134:i16)
                    n182 = Unbundle By Name(w137) -> ("Horizontal"=w130:i32, "Vertical"=w131:i32)
                    n183 = To Long Integer(number=w136) -> (32bit integer=w135:i32)
                    n184 = To Long Integer(number=w134) -> (32bit integer=w133:i32)
                    n185 = Compound Arithmetic op=ADD(invert w135, w130) -> (w129:i32)
                    n186 = Compound Arithmetic op=ADD(invert w133, w131) -> (w128:i32)
                    n187 = Bundle(w129, w128) -> (w127:cluster{i32, i32})  [unwired: 1 in]
                  }
                  frame 1 {
                    n188 = Unbundle By Name(w139) -> ("Left"=w148:i16, "Top"=w146:i16)
                    n189 = Unbundle By Name(w140) -> ("Horizontal"=w143:i32, "Vertical"=w144:i32)
                    n190 = To Long Integer(number=w148) -> (32bit integer=w147:i32)
                    n191 = To Long Integer(number=w146) -> (32bit integer=w145:i32)
                    n192 = Compound Arithmetic op=ADD(invert w147, w143) -> (w142:i32)
                    n193 = Compound Arithmetic op=ADD(invert w145, w144) -> (w141:i32)
                    n194 = Bundle(w142, w141) -> (w138:cluster{i32, i32})  [unwired: 1 in]
                  }
                  frame 3 {
                    n195 = Unbundle By Name(w152) -> ("Left"=w161:i16, "Top"=w159:i16)
                    n196 = Unbundle By Name(w151) -> ("Horizontal"=w153:i32, "Vertical"=w157:i32)
                    n197 = To Long Integer(number=w161) -> (32bit integer=w160:i32)
                    n198 = To Long Integer(number=w159) -> (32bit integer=w158:i32)
                    n199 = local read "Add"() -> (w150:bool)
                    n200 = Compound Arithmetic op=ADD(invert w160, w153) -> (w156:i32)
                    n201 = Compound Arithmetic op=ADD(invert w158, w157) -> (w155:i32)
                    n202 = Bundle(w156, w155) -> (w154:cluster{i32, i32})  [unwired: 1 in]
                    n203 = case shown="True" w150 {
                      tunnel: [w164 w166] -> w162
                      tunnel: w154 -> [w163 w167]
                      tunnel: w149 -> [_ w165]
                      frame False {
                        n204 = Build Array(w163) -> (w164:cluster{i32, i32}[])
                      }
                      frame True {
                        n205 = Build Array (concatenate)(w165, w167) -> (w166:T1[])
                      }
                    }
                  }
                }
              }
              frame True {
                n206 = Unbundle By Name(w168) -> ("Vertical"=w173:i32)
                n207 = Multiply(x=w172, y=w171) -> (x*y=w170:dbl)
                n208 = Subtract(x=w173, y=w170) -> (x-y=w169:dbl)
              }
            }
            n209 = local read "Drawing Mode"() -> (w94:u16)
          }
          event "Image": Mouse Move {
            n210 = event-data() -> ("Coords"=w182:T1)  [unwired: 1 in]
            n211 = case shown="True" w183 {
              tunnel: w182 -> [_ w195]
              tunnel: w181 -> [_ w194]
              tunnel: w180 -> [_ w193]
              tunnel: [_ w192] -> w179
              tunnel: [_ w191] -> w178
              tunnel: w177 -> [_ w190]
              tunnel: [_ w189] -> w176
              tunnel: w175 -> [w186 w188]
              tunnel: [w186 w187] -> w174
              frame False {
              }
              frame True {
                n212 = local read "Rotate"() -> (w196:bool)
                n213 = case shown="False" w196 {
                  tunnel: w195 -> [w201 w276]
                  tunnel: w194 -> [_ w275]
                  tunnel: w193 -> [_ w274]
                  tunnel: [_ w274] -> w192
                  tunnel: [_ w273] -> w191
                  tunnel: w190 -> [w200 _]
                  tunnel: [w199 _] -> w189
                  tunnel: w188 -> [w198 _]
                  tunnel: [w197 _] -> w187
                  frame False {
                    n214 = case shown="5" "Drawing Mode" {
                      tunnel: w201 -> [w213 w224 w235 w246 w259 w270]
                      tunnel: w200 -> [w212 w223 w234 w245 w258 w269]
                      tunnel: [w211 w222 w233 _ w257 w268] -> w199
                      tunnel: w198 -> [_ _ _ w247 _ _]
                      tunnel: [_ _ _ w248 _ _] -> w197
                      frame 0, Default {
                        n215 = Unbundle By Name(w212) -> ("Left"=w210:i16, "Top"=w208:i16)
                        n216 = Unbundle By Name(w213) -> ("Horizontal"=w205:i32, "Vertical"=w206:i32)
                        n217 = To Long Integer(number=w210) -> (32bit integer=w209:i32)
                        n218 = To Long Integer(number=w208) -> (32bit integer=w207:i32)
                        n219 = Compound Arithmetic op=ADD(invert w209, w205) -> (w204:i32)
                        n220 = Compound Arithmetic op=ADD(invert w207, w206) -> (w203:i32)
                        n221 = Bundle(w204, w203) -> (w211:cluster{i32, i32})  [unwired: 1 in]
                      }
                      frame 1 {
                        n222 = Unbundle By Name(w223) -> ("Left"=w221:i16, "Top"=w219:i16)
                        n223 = Unbundle By Name(w224) -> ("Horizontal"=w216:i32, "Vertical"=w217:i32)
                        n224 = To Long Integer(number=w221) -> (32bit integer=w220:i32)
                        n225 = To Long Integer(number=w219) -> (32bit integer=w218:i32)
                        n226 = Compound Arithmetic op=ADD(invert w220, w216) -> (w215:i32)
                        n227 = Compound Arithmetic op=ADD(invert w218, w217) -> (w214:i32)
                        n228 = Bundle(w215, w214) -> (w222:cluster{i32, i32})  [unwired: 1 in]
                      }
                      frame 2 {
                        n229 = Unbundle By Name(w234) -> ("Left"=w232:i16, "Top"=w230:i16)
                        n230 = Unbundle By Name(w235) -> ("Horizontal"=w227:i32, "Vertical"=w228:i32)
                        n231 = To Long Integer(number=w232) -> (32bit integer=w231:i32)
                        n232 = To Long Integer(number=w230) -> (32bit integer=w229:i32)
                        n233 = Compound Arithmetic op=ADD(invert w231, w227) -> (w226:i32)
                        n234 = Compound Arithmetic op=ADD(invert w229, w228) -> (w225:i32)
                        n235 = Bundle(w226, w225) -> (w233:cluster{i32, i32})  [unwired: 1 in]
                      }
                      frame 3 {
                        n236 = Unbundle By Name(w245) -> ("Left"=w236:i16, "Top"=w243:i16)
                        n237 = Unbundle By Name(w246) -> ("Horizontal"=w238:i32, "Vertical"=w241:i32)
                        n238 = To Long Integer(number=w236) -> (32bit integer=w244:i32)
                        n239 = To Long Integer(number=w243) -> (32bit integer=w242:i32)
                        n240 = Compound Arithmetic op=ADD(invert w244, w238) -> (w240:i32)
                        n241 = Compound Arithmetic op=ADD(invert w242, w241) -> (w239:i32)
                        n242 = Bundle(w240, w239) -> (w237:cluster{i32, i32})  [unwired: 1 in]
                        n243 = Build Array (concatenate)(w247, w237) -> (w248:T1[])
                      }
                      frame 4 {
                        n244 = Unbundle By Name(w258) -> ("Left"=w256:i16, "Top"=w254:i16)
                        n245 = Unbundle By Name(w259) -> ("Horizontal"=w251:i32, "Vertical"=w252:i32)
                        n246 = To Long Integer(number=w256) -> (32bit integer=w255:i32)
                        n247 = To Long Integer(number=w254) -> (32bit integer=w253:i32)
                        n248 = Compound Arithmetic op=ADD(invert w255, w251) -> (w250:i32)
                        n249 = Compound Arithmetic op=ADD(invert w253, w252) -> (w249:i32)
                        n250 = Bundle(w250, w249) -> (w257:cluster{i32, i32})  [unwired: 1 in]
                      }
                      frame 5 {
                        n251 = Unbundle By Name(w269) -> ("Left"=w267:i16, "Top"=w265:i16)
                        n252 = Unbundle By Name(w270) -> ("Horizontal"=w262:i32, "Vertical"=w263:i32)
                        n253 = To Long Integer(number=w267) -> (32bit integer=w266:i32)
                        n254 = To Long Integer(number=w265) -> (32bit integer=w264:i32)
                        n255 = Compound Arithmetic op=ADD(invert w266, w262) -> (w261:i32)
                        n256 = Compound Arithmetic op=ADD(invert w264, w263) -> (w260:i32)
                        n257 = Bundle(w261, w260) -> (w268:cluster{i32, i32})  [unwired: 1 in]
                      }
                    }
                  }
                  frame True {
                    n258 = Unbundle By Name(w276) -> ("Vertical"=w272:i32)
                    n259 = Subtract(x=w272, y=w274) -> (x-y=w271:dbl)
                    n260 = Divide(x=w271, y=w275) -> (x/y=w273:dbl)
                  }
                }
              }
            }
          }
          event "Image": Mouse Up {
            n261 = event-data() -> ("Coords"=w283:T1)  [unwired: 1 in]
            n262 = local read "Rotate"() -> (w278:bool)
            n263 = case shown="False" w278 {
              tunnel: w285 -> [w291 _]
              tunnel: w284 -> [w290 _]
              tunnel: w283 -> [w289 _]
              tunnel: w280 -> [w288 _]
              tunnel: w279 -> [_ w1328]
              tunnel: [w286 _] -> w277
              frame False {
                n264 = local read "Drawing Mode"() -> (w287:u16)
                n265 = case shown="5" w287 {
                  selector: w287 -> [w292 w458 w624 w797 w896 w992 w1162]
                  tunnel: w291 -> [w295 w461 w627 w795 w895 w995 w1165]
                  tunnel: w290 -> [w294 w460 w626 _ _ w994 w1164]
                  tunnel: w289 -> [w293 w459 w625 _ _ w993 w1163]
                  tunnel: w288 -> [_ _ _ w796 w894 _ _]
                  tunnel: [_ _ _ w794 _ _ _] -> w286
                  frame 0, Default {
                    n266 = stacked-sequence {
                      seq-local: [w299 _ _ _ _ _] -> [_ w351 _ w413 _ _]
                      seq-local: [w296 _ _ _ _ _] -> [_ w350 _ w388 _ _]
                      seq-local: [w298 _ _ _ _ _] -> [_ w349 _ w412 _ _]
                      seq-local: [w297 _ _ _ _ _] -> [_ w348 _ w387 _ _]
                      tunnel: w295 -> [w308 w345 _ w410 _ _]
                      tunnel: w294 -> [w307 _ _ _ _ _]
                      tunnel: w293 -> [w306 _ _ _ _ _]
                      tunnel: w292 -> [_ _ _ _ _ w457]
                      frame #0 {
                        n267 = Unbundle By Name(w306) -> ("Horizontal"=w314:i32, "Vertical"=w311:i32)
                        n268 = Unbundle By Name(w307) -> ("Horizontal"=w303:i32, "Vertical"=w302:i32)
                        n269 = Unbundle By Name(w308) -> ("Left"=w312:i16, "Top"=w309:i16, "Right"=w301:i16, "Bottom"=w300:i16)
                        n270 = To Long Integer(number=w309) -> (32bit integer=w304:i32)
                        n271 = To Long Integer(number=w312) -> (32bit integer=w305:i32)
                        n272 = To Long Integer(number=w300) -> ()  [unwired: 1 out]
                        n273 = To Long Integer(number=w301) -> ()  [unwired: 1 out]
                        n274 = Compound Arithmetic op=ADD(invert w305, w314) -> (w313:i32)
                        n275 = Compound Arithmetic op=ADD(invert w304, w311) -> (w310:i32)
                        n276 = Max & Min(x=w313, y=w303) -> (max(x,y)=w298:i32, min(x,y)=w299:i32)
                        n277 = Max & Min(x=w310, y=w302) -> (max(x,y)=w297:i32, min(x,y)=w296:i32)
                      }
                      frame #1 {
                        n278 = Unbundle By Name(w345) -> ("Left"=w357:i16, "Top"=w356:i16, "Right"=w355:i16, "Bottom"=w354:i16)
                        n279 = call "2pparameters.vi"("command"="get") -> ("params out"=w343:T6)  [unwired: 1 in]
                        n280 = call "2pparameters.vi"("command"="get") -> ("params out"=w331:T6)  [unwired: 1 in]
                        n281 = To Double Precision Float(number=w357) -> (double precision float=w316:dbl)
                        n282 = To Double Precision Float(number=w356) -> (double precision float=w353:dbl)
                        n283 = To Double Precision Float(number=w355) -> (double precision float=w315:dbl)
                        n284 = To Double Precision Float(number=w354) -> (double precision float=w352:dbl)
                        n285 = Unbundle By Name(w343) -> ("Vx-min Img"=w337:dbl, "VX-max Img"=w342:dbl)
                        n286 = Unbundle By Name(w331) -> ("Vy-max Img"=w329:dbl, "Vy-min Img"=w328:dbl)
                        n287 = call "2pparameters.vi"("command"="get") -> ("params out"=w338:T6)  [unwired: 1 in]
                        n288 = Subtract(x=w337, y=w342) -> (x-y=w341:dbl)
                        n289 = Subtract(x=w316, y=w315) -> (x-y=w347:dbl)
                        n290 = Subtract(x=w353, y=w352) -> (x-y=w346:dbl)
                        n291 = Subtract(x=w329, y=w328) -> (x-y=w327:dbl)
                        n292 = Unbundle By Name(w338) -> ("Vx-min Img"=w333:dbl, "Vy-max Img"=w325:dbl)
                        n293 = Divide(x=w341, y=w347) -> (x/y=w319:dbl)
                        n294 = Divide(x=w327, y=w346) -> (x/y=w318:dbl)
                        n295 = To Double Precision Float(number=w351) -> (double precision float=w320:dbl)
                        n296 = To Double Precision Float(number=w349) -> (double precision float=w335:dbl)
                        n297 = To Double Precision Float(number=w348) -> (double precision float=w326:dbl)
                        n298 = To Double Precision Float(number=w350) -> (double precision float=w317:dbl)
                        n299 = Multiply(x=w320, y=w319) -> (x*y=w336:dbl)
                        n300 = Multiply(x=w319, y=w335) -> (x*y=w334:dbl)
                        n301 = Multiply(x=w326, y=w318) -> (x*y=w324:dbl)
                        n302 = Multiply(x=w318, y=w317) -> (x*y=w323:dbl)
                        n303 = Add(x=w336, y=w333) -> (x+y=w340:dbl)
                        n304 = Add(x=w334, y=w333) -> (x+y=w332:dbl)
                        n305 = Add(x=w325, y=w324) -> (x+y=w322:dbl)
                        n306 = Add(x=w325, y=w323) -> (x+y=w321:dbl)
                        n307 = local write "Vy-min"(w322) -> ()
                        n308 = local write "Vx-min"(w340) -> ()
                        n309 = local write "Vy-max"(w321) -> ()
                        n310 = local write "Vx-max"(w332) -> ()
                      }
                      frame #2 {
                        n311 = local read "Vy-max"() -> (w383:dbl)
                        n312 = local read "Vy-min"() -> (w384:dbl)
                        n313 = local read "Vx-max"() -> (w381:dbl)
                        n314 = local read "Vx-min"() -> (w382:dbl)
                        n315 = call "2pparameters.vi"("command"="get") -> ("params out"=w371:T6)  [unwired: 1 in]
                        n316 = Unbundle By Name(w371) -> ("VX-max Img"=w373:dbl, "Vx-min Img"=w374:dbl, "Vy-max Img"=w375:dbl, "Vy-min Img"=w376:dbl, "Angle Img"=w366:dbl)
                        n317 = Add(x=w373, y=w374) -> (x+y=w377:dbl)
                        n318 = Add(x=w375, y=w376) -> (x+y=w380:dbl)
                        n319 = Divide(x=w377, y=2.0) -> (x/y=w361:dbl)
                        n320 = Subtract(x=w381, y=w361) -> (x-y=w370:dbl)
                        n321 = Subtract(x=w382, y=w361) -> (x-y=w369:dbl)
                        n322 = Divide(x=w380, y=2.0) -> (x/y=w360:dbl)
                        n323 = Subtract(x=w384, y=w360) -> (x-y=w367:dbl)
                        n324 = Subtract(x=w383, y=w360) -> (x-y=w368:dbl)
                        n325 = script code="Xic=(ximax+ximin)./2;\nYic=(yimax+yimin)./2;\nXicrot=Xic.*cos(pi/180.*phi)+Yic.*sin(pi./180.*phi);\nYicrot=-Xic.*sin(pi./180.*phi)+Yic.*cos(pi./180.*phi);\nxirmax=ximax-Xic+Xicrot;\nxirmin=ximin-Xic+Xicrot;\nyirmax=yimax-Yic+Yicrot;\nyirmin=yimin-Yic+Yicrot;"("ximax"=w370, "ximin"=w369, "yimax"=w368, "yimin"=w367, "phi"=w366) -> ("xirmax"=w365:dbl, "xirmin"=w364:dbl, "yirmax"=w363:dbl, "yirmin"=w362:dbl)  [unwired: 1 in, 1 out]
                        n326 = Add(x=w362, y=w360) -> (x+y=w358:dbl)
                        n327 = Add(x=w363, y=w360) -> (x+y=w359:dbl)
                        n328 = Add(x=w364, y=w361) -> (x+y=w386:dbl)
                        n329 = Add(x=w365, y=w361) -> (x+y=w385:dbl)
                        n330 = local write "Vy-max"(w359) -> ()
                        n331 = local write "Vx-min"(w386) -> ()
                        n332 = local write "Vx-max"(w385) -> ()
                        n333 = local write "Vy-min"(w358) -> ()
                      }
                      frame #3 {
                        n334 = Unbundle By Name(w410) -> ("Left"=w419:i16, "Top"=w418:i16, "Right"=w417:i16, "Bottom"=w416:i16)
                        n335 = To Double Precision Float(number=w419) -> (double precision float=w404:dbl)
                        n336 = To Double Precision Float(number=w418) -> (double precision float=w415:dbl)
                        n337 = To Double Precision Float(number=w417) -> (double precision float=w403:dbl)
                        n338 = To Double Precision Float(number=w416) -> (double precision float=w414:dbl)
                        n339 = call "2pparameters.vi"("command"="get") -> ("params out"=w409:T6)  [unwired: 1 in]
                        n340 = Subtract(x=w404, y=w403) -> (x-y=w411:dbl)
                        n341 = Subtract(x=w415, y=w414) -> (x-y=w389:dbl)
                        n342 = Unbundle By Name(w409) -> ("Xpixels Img"=w401:i32, "Ypixels Img"=w400:i32)
                        n343 = To Double Precision Float(number=w413) -> (double precision float=w407:dbl)
                        n344 = To Double Precision Float(number=w412) -> (double precision float=w402:dbl)
                        n345 = To Double Precision Float(number=w388) -> (double precision float=w406:dbl)
                        n346 = To Double Precision Float(number=w387) -> (double precision float=w405:dbl)
                        n347 = To Double Precision Float(number=w401) -> (double precision float=w397:dbl)
                        n348 = To Double Precision Float(number=w400) -> (double precision float=w395:dbl)
                        n349 = Subtract(x=w406, y=w405) -> (x-y=w396:dbl)
                        n350 = Subtract(x=w407, y=w402) -> (x-y=w399:dbl)
                        n351 = Divide(x=w399, y=w411) -> (x/y=w398:dbl)
                        n352 = Divide(x=w396, y=w389) -> (x/y=w394:dbl)
                        n353 = Multiply(x=w398, y=w397) -> (x*y=w392:dbl)
                        n354 = Multiply(x=w395, y=w394) -> (x*y=w393:dbl)
                        n355 = To Long Integer(number=w392) -> (32bit integer=w391:i32)
                        n356 = To Long Integer(number=w393) -> (32bit integer=w390:i32)
                        n357 = local write "Xpixels"(w391) -> ()
                        n358 = local write "Ypixels"(w390) -> ()
                      }
                      frame #4 {
                        n359 = local read "square pixels"() -> (w420:bool)
                        n360 = case shown="True" w420 {
                          frame False {
                            n361 = local read "square matrix"() -> (w421:bool)
                            n362 = case shown="True" w421 {
                              frame False {
                              }
                              frame True {
                                n363 = local read "Xpixels"() -> (w424:i32)
                                n364 = local read "Ypixels"() -> (w423:i32)
                                n365 = Max & Min(x=w424, y=w423) -> (max(x,y)=w422:i32)  [unwired: 1 out]
                                n366 = local write "Ypixels"(w422) -> ()
                                n367 = local write "Xpixels"(w422) -> ()
                              }
                            }
                          }
                          frame True {
                            n368 = local read "square matrix"() -> (w425:bool)
                            n369 = case shown="False" w425 {
                              frame False {
                                n370 = local read "Vy-min"() -> (w435:dbl)
                                n371 = local read "Vx-max"() -> (w439:dbl)
                                n372 = local read "Vx-min"() -> (w438:dbl)
                                n373 = local read "Vy-max"() -> (w434:dbl)
                                n374 = Subtract(x=w434, y=w435) -> (x-y=w436:dbl)
                                n375 = Subtract(x=w439, y=w438) -> (x-y=w437:dbl)
                                n376 = Absolute Value(x=w436) -> (abs(x)=w427:dbl)
                                n377 = Absolute Value(x=w437) -> (abs(x)=w428:dbl)
                                n378 = local read "Xpixels"() -> (w432:i32)
                                n379 = Divide(x=w428, y=w427) -> (x/y=w433:dbl)
                                n380 = local read "Ypixels"() -> (w429:i32)
                                n381 = Greater Or Equal?(x=w428, y=w427) -> (x >= y?=w426:bool)
                                n382 = case shown="False" w426 {
                                tunnel: w433 -> [w444 w447]
                                tunnel: w432 -> [w441 _]
                                tunnel: [w441 w446] -> w431
                                tunnel: [w440 w445] -> w430
                                tunnel: w429 -> [_ w445]
                                frame False {
                                n383 = To Double Precision Float(number=w441) -> (double precision float=w443:dbl)
                                n384 = Divide(x=w443, y=w444) -> (x/y=w442:dbl)
                                n385 = To Long Integer(number=w442) -> (32bit integer=w440:i32)
                                }
                                frame True {
                                n386 = To Double Precision Float(number=w445) -> (double precision float=w449:dbl)
                                n387 = Multiply(x=w449, y=w447) -> (x*y=w448:dbl)
                                n388 = To Long Integer(number=w448) -> (32bit integer=w446:i32)
                                }
                                }
                                n389 = local write "Xpixels"(w431) -> ()
                                n390 = local write "Ypixels"(w430) -> ()
                              }
                              frame True {
                              }
                            }
                          }
                        }
                      }
                      frame #5 {
                        n391 = local read "Vy-min"() -> (w450:dbl)
                        n392 = local read "Vx-max"() -> (w453:dbl)
                        n393 = local read "Vx-min"() -> (w452:dbl)
                        n394 = local read "Vy-max"() -> (w451:dbl)
                        n395 = local read "Ypixels"() -> (w455:i32)
                        n396 = local read "Xpixels"() -> (w456:i32)
                        n397 = local read "Angle"() -> (w454:dbl)
                        n398 = call "ScanningWaveform_v4.vi"("Vy-min"=w450, "Vy-max"=w451, "yPixels/tPixels"=w455, "xPixels/rPixels"=w456, "Vx-min"=w452, "Vx-max"=w453, "Drawing Mode"=w457, "Angle"=w454) -> ()  [unwired: 8 in, 4 out]
                      }
                    }
                  }
                  frame 1 {
                    n399 = stacked-sequence {
                      seq-local: [w465 _ _ _ _ _] -> [_ w517 _ w579 _ _]
                      seq-local: [w462 _ _ _ _ _] -> [_ w516 _ w554 _ _]
                      seq-local: [w464 _ _ _ _ _] -> [_ w515 _ w578 _ _]
                      seq-local: [w463 _ _ _ _ _] -> [_ w514 _ w553 _ _]
                      tunnel: w461 -> [w474 w511 _ w576 _ _]
                      tunnel: w460 -> [w473 _ _ _ _ _]
                      tunnel: w459 -> [w472 _ _ _ _ _]
                      tunnel: w458 -> [_ _ _ _ _ w623]
                      frame #0 {
                        n400 = Unbundle By Name(w472) -> ("Horizontal"=w480:i32, "Vertical"=w477:i32)
                        n401 = Unbundle By Name(w473) -> ("Horizontal"=w469:i32, "Vertical"=w468:i32)
                        n402 = Unbundle By Name(w474) -> ("Left"=w478:i16, "Top"=w475:i16, "Right"=w467:i16, "Bottom"=w466:i16)
                        n403 = To Long Integer(number=w475) -> (32bit integer=w470:i32)
                        n404 = To Long Integer(number=w478) -> (32bit integer=w471:i32)
                        n405 = To Long Integer(number=w466) -> ()  [unwired: 1 out]
                        n406 = To Long Integer(number=w467) -> ()  [unwired: 1 out]
                        n407 = Compound Arithmetic op=ADD(invert w471, w480) -> (w479:i32)
                        n408 = Compound Arithmetic op=ADD(invert w470, w477) -> (w476:i32)
                        n409 = Max & Min(x=w479, y=w469) -> (max(x,y)=w464:i32, min(x,y)=w465:i32)
                        n410 = Max & Min(x=w476, y=w468) -> (max(x,y)=w463:i32, min(x,y)=w462:i32)
                      }
                      frame #1 {
                        n411 = Unbundle By Name(w511) -> ("Left"=w523:i16, "Top"=w522:i16, "Right"=w521:i16, "Bottom"=w520:i16)
                        n412 = call "2pparameters.vi"("command"="get") -> ("params out"=w509:T6)  [unwired: 1 in]
                        n413 = call "2pparameters.vi"("command"="get") -> ("params out"=w497:T6)  [unwired: 1 in]
                        n414 = To Double Precision Float(number=w523) -> (double precision float=w482:dbl)
                        n415 = To Double Precision Float(number=w522) -> (double precision float=w519:dbl)
                        n416 = To Double Precision Float(number=w521) -> (double precision float=w481:dbl)
                        n417 = To Double Precision Float(number=w520) -> (double precision float=w518:dbl)
                        n418 = Unbundle By Name(w509) -> ("Vx-min Img"=w503:dbl, "VX-max Img"=w508:dbl)
                        n419 = Unbundle By Name(w497) -> ("Vy-max Img"=w495:dbl, "Vy-min Img"=w494:dbl)
                        n420 = call "2pparameters.vi"("command"="get") -> ("params out"=w504:T6)  [unwired: 1 in]
                        n421 = Subtract(x=w503, y=w508) -> (x-y=w507:dbl)
                        n422 = Subtract(x=w482, y=w481) -> (x-y=w513:dbl)
                        n423 = Subtract(x=w519, y=w518) -> (x-y=w512:dbl)
                        n424 = Subtract(x=w495, y=w494) -> (x-y=w493:dbl)
                        n425 = Unbundle By Name(w504) -> ("Vx-min Img"=w499:dbl, "Vy-max Img"=w491:dbl)
                        n426 = Divide(x=w507, y=w513) -> (x/y=w485:dbl)
                        n427 = Divide(x=w493, y=w512) -> (x/y=w484:dbl)
                        n428 = To Double Precision Float(number=w517) -> (double precision float=w486:dbl)
                        n429 = To Double Precision Float(number=w515) -> (double precision float=w501:dbl)
                        n430 = To Double Precision Float(number=w514) -> (double precision float=w492:dbl)
                        n431 = To Double Precision Float(number=w516) -> (double precision float=w483:dbl)
                        n432 = Multiply(x=w486, y=w485) -> (x*y=w502:dbl)
                        n433 = Multiply(x=w485, y=w501) -> (x*y=w500:dbl)
                        n434 = Multiply(x=w492, y=w484) -> (x*y=w490:dbl)
                        n435 = Multiply(x=w484, y=w483) -> (x*y=w489:dbl)
                        n436 = Add(x=w502, y=w499) -> (x+y=w506:dbl)
                        n437 = Add(x=w500, y=w499) -> (x+y=w498:dbl)
                        n438 = Add(x=w491, y=w490) -> (x+y=w488:dbl)
                        n439 = Add(x=w491, y=w489) -> (x+y=w487:dbl)
                        n440 = local write "Vy-min"(w488) -> ()
                        n441 = local write "Vx-min"(w506) -> ()
                        n442 = local write "Vy-max"(w487) -> ()
                        n443 = local write "Vx-max"(w498) -> ()
                      }
                      frame #2 {
                        n444 = local read "Vy-max"() -> (w549:dbl)
                        n445 = local read "Vy-min"() -> (w550:dbl)
                        n446 = local read "Vx-max"() -> (w547:dbl)
                        n447 = local read "Vx-min"() -> (w548:dbl)
                        n448 = call "2pparameters.vi"("command"="get") -> ("params out"=w537:T6)  [unwired: 1 in]
                        n449 = Unbundle By Name(w537) -> ("VX-max Img"=w539:dbl, "Vx-min Img"=w540:dbl, "Vy-max Img"=w541:dbl, "Vy-min Img"=w542:dbl, "Angle Img"=w532:dbl)
                        n450 = Add(x=w539, y=w540) -> (x+y=w543:dbl)
                        n451 = Add(x=w541, y=w542) -> (x+y=w546:dbl)
                        n452 = Divide(x=w543, y=2.0) -> (x/y=w527:dbl)
                        n453 = Subtract(x=w547, y=w527) -> (x-y=w536:dbl)
                        n454 = Subtract(x=w548, y=w527) -> (x-y=w535:dbl)
                        n455 = Divide(x=w546, y=2.0) -> (x/y=w526:dbl)
                        n456 = Subtract(x=w550, y=w526) -> (x-y=w533:dbl)
                        n457 = Subtract(x=w549, y=w526) -> (x-y=w534:dbl)
                        n458 = script code="Xic=(ximax+ximin)./2;\nYic=(yimax+yimin)./2;\nXicrot=Xic.*cos(pi/180.*phi)+Yic.*sin(pi./180.*phi);\nYicrot=-Xic.*sin(pi./180.*phi)+Yic.*cos(pi./180.*phi);\nxirmax=ximax-Xic+Xicrot;\nxirmin=ximin-Xic+Xicrot;\nyirmax=yimax-Yic+Yicrot;\nyirmin=yimin-Yic+Yicrot;"("ximax"=w536, "ximin"=w535, "yimax"=w534, "yimin"=w533, "phi"=w532) -> ("xirmax"=w531:dbl, "xirmin"=w530:dbl, "yirmax"=w529:dbl, "yirmin"=w528:dbl)  [unwired: 1 in, 1 out]
                        n459 = Add(x=w528, y=w526) -> (x+y=w524:dbl)
                        n460 = Add(x=w529, y=w526) -> (x+y=w525:dbl)
                        n461 = Add(x=w530, y=w527) -> (x+y=w552:dbl)
                        n462 = Add(x=w531, y=w527) -> (x+y=w551:dbl)
                        n463 = local write "Vy-max"(w525) -> ()
                        n464 = local write "Vx-min"(w552) -> ()
                        n465 = local write "Vx-max"(w551) -> ()
                        n466 = local write "Vy-min"(w524) -> ()
                      }
                      frame #3 {
                        n467 = Unbundle By Name(w576) -> ("Left"=w585:i16, "Top"=w584:i16, "Right"=w583:i16, "Bottom"=w582:i16)
                        n468 = To Double Precision Float(number=w585) -> (double precision float=w570:dbl)
                        n469 = To Double Precision Float(number=w584) -> (double precision float=w581:dbl)
                        n470 = To Double Precision Float(number=w583) -> (double precision float=w569:dbl)
                        n471 = To Double Precision Float(number=w582) -> (double precision float=w580:dbl)
                        n472 = call "2pparameters.vi"("command"="get") -> ("params out"=w575:T6)  [unwired: 1 in]
                        n473 = Subtract(x=w570, y=w569) -> (x-y=w577:dbl)
                        n474 = Subtract(x=w581, y=w580) -> (x-y=w555:dbl)
                        n475 = Unbundle By Name(w575) -> ("Xpixels Img"=w567:i32, "Ypixels Img"=w566:i32)
                        n476 = To Double Precision Float(number=w579) -> (double precision float=w573:dbl)
                        n477 = To Double Precision Float(number=w578) -> (double precision float=w568:dbl)
                        n478 = To Double Precision Float(number=w554) -> (double precision float=w572:dbl)
                        n479 = To Double Precision Float(number=w553) -> (double precision float=w571:dbl)
                        n480 = To Double Precision Float(number=w567) -> (double precision float=w563:dbl)
                        n481 = To Double Precision Float(number=w566) -> (double precision float=w561:dbl)
                        n482 = Subtract(x=w572, y=w571) -> (x-y=w562:dbl)
                        n483 = Subtract(x=w573, y=w568) -> (x-y=w565:dbl)
                        n484 = Divide(x=w565, y=w577) -> (x/y=w564:dbl)
                        n485 = Divide(x=w562, y=w555) -> (x/y=w560:dbl)
                        n486 = Multiply(x=w564, y=w563) -> (x*y=w558:dbl)
                        n487 = Multiply(x=w561, y=w560) -> (x*y=w559:dbl)
                        n488 = To Long Integer(number=w558) -> (32bit integer=w557:i32)
                        n489 = To Long Integer(number=w559) -> (32bit integer=w556:i32)
                        n490 = local write "Xpixels"(w557) -> ()
                        n491 = local write "Ypixels"(w556) -> ()
                      }
                      frame #4 {
                        n492 = local read "square pixels"() -> (w586:bool)
                        n493 = case shown="True" w586 {
                          frame False {
                            n494 = local read "square matrix"() -> (w587:bool)
                            n495 = case shown="True" w587 {
                              frame False {
                              }
                              frame True {
                                n496 = local read "Xpixels"() -> (w590:i32)
                                n497 = local read "Ypixels"() -> (w589:i32)
                                n498 = Max & Min(x=w590, y=w589) -> (max(x,y)=w588:i32)  [unwired: 1 out]
                                n499 = local write "Ypixels"(w588) -> ()
                                n500 = local write "Xpixels"(w588) -> ()
                              }
                            }
                          }
                          frame True {
                            n501 = local read "square matrix"() -> (w591:bool)
                            n502 = case shown="False" w591 {
                              frame False {
                                n503 = local read "Vy-min"() -> (w601:dbl)
                                n504 = local read "Vx-max"() -> (w605:dbl)
                                n505 = local read "Vx-min"() -> (w604:dbl)
                                n506 = local read "Vy-max"() -> (w600:dbl)
                                n507 = Subtract(x=w600, y=w601) -> (x-y=w602:dbl)
                                n508 = Subtract(x=w605, y=w604) -> (x-y=w603:dbl)
                                n509 = Absolute Value(x=w602) -> (abs(x)=w593:dbl)
                                n510 = Absolute Value(x=w603) -> (abs(x)=w594:dbl)
                                n511 = local read "Xpixels"() -> (w598:i32)
                                n512 = Divide(x=w594, y=w593) -> (x/y=w599:dbl)
                                n513 = local read "Ypixels"() -> (w595:i32)
                                n514 = Greater Or Equal?(x=w594, y=w593) -> (x >= y?=w592:bool)
                                n515 = case shown="False" w592 {
                                tunnel: w599 -> [w610 w613]
                                tunnel: w598 -> [w607 _]
                                tunnel: [w607 w612] -> w597
                                tunnel: [w606 w611] -> w596
                                tunnel: w595 -> [_ w611]
                                frame False {
                                n516 = To Double Precision Float(number=w607) -> (double precision float=w609:dbl)
                                n517 = Divide(x=w609, y=w610) -> (x/y=w608:dbl)
                                n518 = To Long Integer(number=w608) -> (32bit integer=w606:i32)
                                }
                                frame True {
                                n519 = To Double Precision Float(number=w611) -> (double precision float=w615:dbl)
                                n520 = Multiply(x=w615, y=w613) -> (x*y=w614:dbl)
                                n521 = To Long Integer(number=w614) -> (32bit integer=w612:i32)
                                }
                                }
                                n522 = local write "Xpixels"(w597) -> ()
                                n523 = local write "Ypixels"(w596) -> ()
                              }
                              frame True {
                              }
                            }
                          }
                        }
                      }
                      frame #5 {
                        n524 = local read "Vy-min"() -> (w616:dbl)
                        n525 = local read "Vx-max"() -> (w619:dbl)
                        n526 = local read "Vx-min"() -> (w618:dbl)
                        n527 = local read "Vy-max"() -> (w617:dbl)
                        n528 = local read "Ypixels"() -> (w621:i32)
                        n529 = local read "Xpixels"() -> (w622:i32)
                        n530 = local read "Angle"() -> (w620:dbl)
                        n531 = call "ScanningWaveform_v4.vi"("Vy-min"=w616, "Vy-max"=w617, "yPixels/tPixels"=w621, "xPixels/rPixels"=w622, "Vx-min"=w618, "Vx-max"=w619, "Drawing Mode"=w623, "Angle"=w620) -> ()  [unwired: 8 in, 4 out]
                      }
                    }
                  }
                  frame 2 {
                    n532 = stacked-sequence {
                      seq-local: [w638 _ _ _ _ _] -> [_ w686 _ w748 _ _]
                      seq-local: [w635 _ _ _ _ _] -> [_ w685 _ w723 _ _]
                      seq-local: [w637 _ _ _ _ _] -> [_ w684 _ w747 _ _]
                      seq-local: [w636 _ _ _ _ _] -> [_ w683 _ w722 _ _]
                      tunnel: w627 -> [w645 w680 _ w745 _ _]
                      tunnel: w626 -> [w644 _ _ _ _ _]
                      tunnel: w625 -> [w643 _ _ _ _ _]
                      tunnel: w624 -> [_ _ _ _ _ w793]
                      frame #0 {
                        w632 = 2 ("value")
                        n533 = Unbundle By Name(w643) -> ("Horizontal"=w649:i32, "Vertical"=w647:i32)
                        n534 = Unbundle By Name(w644) -> ("Horizontal"=w640:i32, "Vertical"=w639:i32)
                        n535 = Unbundle By Name(w645) -> ("Left"=w648:i16, "Top"=w646:i16)
                        n536 = To Long Integer(number=w646) -> (32bit integer=w641:i32)
                        n537 = To Long Integer(number=w648) -> (32bit integer=w642:i32)
                        n538 = Compound Arithmetic op=MULTIPLY(w640, w632) -> (w634:i32)
                        n539 = Compound Arithmetic op=MULTIPLY(w639, w632) -> (w633:i32)
                        n540 = Compound Arithmetic op=ADD(invert w642, w649) -> (w629:i32)
                        n541 = Compound Arithmetic op=ADD(invert w641, w647) -> (w628:i32)
                        n542 = Compound Arithmetic op=ADD(invert w629, w634) -> (w631:i32)
                        n543 = Compound Arithmetic op=ADD(invert w628, w633) -> (w630:i32)
                        n544 = Max & Min(x=w629, y=w631) -> (max(x,y)=w637:i32, min(x,y)=w638:i32)
                        n545 = Max & Min(x=w628, y=w630) -> (max(x,y)=w636:i32, min(x,y)=w635:i32)
                      }
                      frame #1 {
                        n546 = Unbundle By Name(w680) -> ("Left"=w692:i16, "Top"=w691:i16, "Right"=w690:i16, "Bottom"=w689:i16)
                        n547 = call "2pparameters.vi"("command"="get") -> ("params out"=w678:T6)  [unwired: 1 in]
                        n548 = call "2pparameters.vi"("command"="get") -> ("params out"=w666:T6)  [unwired: 1 in]
                        n549 = To Double Precision Float(number=w692) -> (double precision float=w651:dbl)
                        n550 = To Double Precision Float(number=w691) -> (double precision float=w688:dbl)
                        n551 = To Double Precision Float(number=w690) -> (double precision float=w650:dbl)
                        n552 = To Double Precision Float(number=w689) -> (double precision float=w687:dbl)
                        n553 = Unbundle By Name(w678) -> ("Vx-min Img"=w672:dbl, "VX-max Img"=w677:dbl)
                        n554 = Unbundle By Name(w666) -> ("Vy-max Img"=w664:dbl, "Vy-min Img"=w663:dbl)
                        n555 = call "2pparameters.vi"("command"="get") -> ("params out"=w673:T6)  [unwired: 1 in]
                        n556 = Subtract(x=w672, y=w677) -> (x-y=w676:dbl)
                        n557 = Subtract(x=w651, y=w650) -> (x-y=w682:dbl)
                        n558 = Subtract(x=w688, y=w687) -> (x-y=w681:dbl)
                        n559 = Subtract(x=w664, y=w663) -> (x-y=w662:dbl)
                        n560 = Unbundle By Name(w673) -> ("Vx-min Img"=w668:dbl, "Vy-max Img"=w660:dbl)
                        n561 = Divide(x=w676, y=w682) -> (x/y=w654:dbl)
                        n562 = Divide(x=w662, y=w681) -> (x/y=w653:dbl)
                        n563 = To Double Precision Float(number=w686) -> (double precision float=w655:dbl)
                        n564 = To Double Precision Float(number=w684) -> (double precision float=w670:dbl)
                        n565 = To Double Precision Float(number=w683) -> (double precision float=w661:dbl)
                        n566 = To Double Precision Float(number=w685) -> (double precision float=w652:dbl)
                        n567 = Multiply(x=w655, y=w654) -> (x*y=w671:dbl)
                        n568 = Multiply(x=w654, y=w670) -> (x*y=w669:dbl)
                        n569 = Multiply(x=w661, y=w653) -> (x*y=w659:dbl)
                        n570 = Multiply(x=w653, y=w652) -> (x*y=w658:dbl)
                        n571 = Add(x=w671, y=w668) -> (x+y=w675:dbl)
                        n572 = Add(x=w669, y=w668) -> (x+y=w667:dbl)
                        n573 = Add(x=w660, y=w659) -> (x+y=w657:dbl)
                        n574 = Add(x=w660, y=w658) -> (x+y=w656:dbl)
                        n575 = local write "Vy-min"(w657) -> ()
                        n576 = local write "Vx-min"(w675) -> ()
                        n577 = local write "Vy-max"(w656) -> ()
                        n578 = local write "Vx-max"(w667) -> ()
                      }
                      frame #2 {
                        n579 = local read "Vy-max"() -> (w718:dbl)
                        n580 = local read "Vy-min"() -> (w719:dbl)
                        n581 = local read "Vx-max"() -> (w716:dbl)
                        n582 = local read "Vx-min"() -> (w717:dbl)
                        n583 = call "2pparameters.vi"("command"="get") -> ("params out"=w706:T6)  [unwired: 1 in]
                        n584 = Unbundle By Name(w706) -> ("VX-max Img"=w708:dbl, "Vx-min Img"=w709:dbl, "Vy-max Img"=w710:dbl, "Vy-min Img"=w711:dbl, "Angle Img"=w701:dbl)
                        n585 = Add(x=w708, y=w709) -> (x+y=w712:dbl)
                        n586 = Add(x=w710, y=w711) -> (x+y=w715:dbl)
                        n587 = Divide(x=w712, y=2.0) -> (x/y=w696:dbl)
                        n588 = Subtract(x=w716, y=w696) -> (x-y=w705:dbl)
                        n589 = Subtract(x=w717, y=w696) -> (x-y=w704:dbl)
                        n590 = Divide(x=w715, y=2.0) -> (x/y=w695:dbl)
                        n591 = Subtract(x=w719, y=w695) -> (x-y=w702:dbl)
                        n592 = Subtract(x=w718, y=w695) -> (x-y=w703:dbl)
                        n593 = script code="Xic=(ximax+ximin)./2;\nYic=(yimax+yimin)./2;\nXicrot=Xic.*cos(pi/180.*phi)+Yic.*sin(pi./180.*phi);\nYicrot=-Xic.*sin(pi./180.*phi)+Yic.*cos(pi./180.*phi);\nxirmax=ximax-Xic+Xicrot;\nxirmin=ximin-Xic+Xicrot;\nyirmax=yimax-Yic+Yicrot;\nyirmin=yimin-Yic+Yicrot;"("ximax"=w705, "ximin"=w704, "yimax"=w703, "yimin"=w702, "phi"=w701) -> ("xirmax"=w700:dbl, "xirmin"=w699:dbl, "yirmax"=w698:dbl, "yirmin"=w697:dbl)  [unwired: 1 in, 1 out]
                        n594 = Add(x=w697, y=w695) -> (x+y=w693:dbl)
                        n595 = Add(x=w698, y=w695) -> (x+y=w694:dbl)
                        n596 = Add(x=w699, y=w696) -> (x+y=w721:dbl)
                        n597 = Add(x=w700, y=w696) -> (x+y=w720:dbl)
                        n598 = local write "Vy-max"(w694) -> ()
                        n599 = local write "Vx-min"(w721) -> ()
                        n600 = local write "Vx-max"(w720) -> ()
                        n601 = local write "Vy-min"(w693) -> ()
                      }
                      frame #3 {
                        n602 = Unbundle By Name(w745) -> ("Left"=w754:i16, "Top"=w753:i16, "Right"=w752:i16, "Bottom"=w751:i16)
                        n603 = To Double Precision Float(number=w754) -> (double precision float=w739:dbl)
                        n604 = To Double Precision Float(number=w753) -> (double precision float=w750:dbl)
                        n605 = To Double Precision Float(number=w752) -> (double precision float=w738:dbl)
                        n606 = To Double Precision Float(number=w751) -> (double precision float=w749:dbl)
                        n607 = call "2pparameters.vi"("command"="get") -> ("params out"=w744:T6)  [unwired: 1 in]
                        n608 = Subtract(x=w739, y=w738) -> (x-y=w746:dbl)
                        n609 = Subtract(x=w750, y=w749) -> (x-y=w724:dbl)
                        n610 = Unbundle By Name(w744) -> ("Xpixels Img"=w736:i32, "Ypixels Img"=w735:i32)
                        n611 = To Double Precision Float(number=w748) -> (double precision float=w742:dbl)
                        n612 = To Double Precision Float(number=w747) -> (double precision float=w737:dbl)
                        n613 = To Double Precision Float(number=w723) -> (double precision float=w741:dbl)
                        n614 = To Double Precision Float(number=w722) -> (double precision float=w740:dbl)
                        n615 = To Double Precision Float(number=w736) -> (double precision float=w732:dbl)
                        n616 = To Double Precision Float(number=w735) -> (double precision float=w730:dbl)
                        n617 = Subtract(x=w741, y=w740) -> (x-y=w731:dbl)
                        n618 = Subtract(x=w742, y=w737) -> (x-y=w734:dbl)
                        n619 = Divide(x=w734, y=w746) -> (x/y=w733:dbl)
                        n620 = Divide(x=w731, y=w724) -> (x/y=w729:dbl)
                        n621 = Multiply(x=w733, y=w732) -> (x*y=w727:dbl)
                        n622 = Multiply(x=w730, y=w729) -> (x*y=w728:dbl)
                        n623 = To Long Integer(number=w727) -> (32bit integer=w726:i32)
                        n624 = To Long Integer(number=w728) -> (32bit integer=w725:i32)
                        n625 = local write "Xpixels"(w726) -> ()
                        n626 = local write "Ypixels"(w725) -> ()
                      }
                      frame #4 {
                        n627 = local read "square pixels"() -> (w755:bool)
                        n628 = case shown="True" w755 {
                          frame False {
                            n629 = local read "square matrix"() -> (w756:bool)
                            n630 = case shown="True" w756 {
                              frame False {
                              }
                              frame True {
                                n631 = local read "Xpixels"() -> (w759:i32)
                                n632 = local read "Ypixels"() -> (w758:i32)
                                n633 = Max & Min(x=w759, y=w758) -> (max(x,y)=w757:i32)  [unwired: 1 out]
                                n634 = local write "Ypixels"(w757) -> ()
                                n635 = local write "Xpixels"(w757) -> ()
                              }
                            }
                          }
                          frame True {
                            n636 = local read "square matrix"() -> (w760:bool)
                            n637 = case shown="False" w760 {
                              frame False {
                                n638 = local read "Vy-min"() -> (w770:dbl)
                                n639 = local read "Vx-max"() -> (w774:dbl)
                                n640 = local read "Vx-min"() -> (w773:dbl)
                                n641 = local read "Vy-max"() -> (w769:dbl)
                                n642 = Subtract(x=w769, y=w770) -> (x-y=w771:dbl)
                                n643 = Subtract(x=w774, y=w773) -> (x-y=w772:dbl)
                                n644 = Absolute Value(x=w771) -> (abs(x)=w762:dbl)
                                n645 = Absolute Value(x=w772) -> (abs(x)=w763:dbl)
                                n646 = local read "Xpixels"() -> (w767:i32)
                                n647 = Divide(x=w763, y=w762) -> (x/y=w768:dbl)
                                n648 = local read "Ypixels"() -> (w764:i32)
                                n649 = Greater Or Equal?(x=w763, y=w762) -> (x >= y?=w761:bool)
                                n650 = case shown="False" w761 {
                                tunnel: w768 -> [w779 w782]
                                tunnel: w767 -> [w776 _]
                                tunnel: [w776 w781] -> w766
                                tunnel: [w775 w780] -> w765
                                tunnel: w764 -> [_ w780]
                                frame False {
                                n651 = To Double Precision Float(number=w776) -> (double precision float=w778:dbl)
                                n652 = Divide(x=w778, y=w779) -> (x/y=w777:dbl)
                                n653 = To Long Integer(number=w777) -> (32bit integer=w775:i32)
                                }
                                frame True {
                                n654 = To Double Precision Float(number=w780) -> (double precision float=w784:dbl)
                                n655 = Multiply(x=w784, y=w782) -> (x*y=w783:dbl)
                                n656 = To Long Integer(number=w783) -> (32bit integer=w781:i32)
                                }
                                }
                                n657 = local write "Xpixels"(w766) -> ()
                                n658 = local write "Ypixels"(w765) -> ()
                              }
                              frame True {
                              }
                            }
                          }
                        }
                      }
                      frame #5 {
                        n659 = local read "Vy-min"() -> (w786:dbl)
                        n660 = local read "Vx-max"() -> (w789:dbl)
                        n661 = local read "Vx-min"() -> (w788:dbl)
                        n662 = local read "Vy-max"() -> (w787:dbl)
                        n663 = local read "Ypixels"() -> (w791:i32)
                        n664 = local read "Xpixels"() -> (w792:i32)
                        n665 = local read "Angle"() -> (w790:dbl)
                        n666 = call "ScanningWaveform_v4.vi"("Vy-min"=w786, "Vy-max"=w787, "yPixels/tPixels"=w791, "xPixels/rPixels"=w792, "Vx-min"=w788, "Vx-max"=w789, "Drawing Mode"=w793, "Angle"=w790, "points in ellipse"=100.0) -> ()  [unwired: 7 in, 4 out]
                      }
                    }
                  }
                  frame 3 {
                    n667 = stacked-sequence {
                      seq-local: [w801 _ _ _] -> [_ w812 _ _]
                      seq-local: [w800 _ _ _] -> [_ w811 _ _]
                      seq-local: [w802 _ _ _] -> [_ w810 _ _]
                      seq-local: [w799 _ _ _] -> [_ w809 _ _]
                      tunnel: w797 -> [_ _ _ w881]
                      tunnel: w796 -> [w798 _ _ w880]
                      tunnel: w795 -> [_ w808 _ _]
                      tunnel: [w798 _ _ _] -> w794
                      frame #0 {
                        n668 = Array Max & Min(array=w798) -> (max value=w805:T1, min value=w804:T1)  [unwired: 2 out]
                        n669 = Unbundle By Name(w805) -> ("Horizontal"=w802:i32)
                        n670 = Unbundle By Name(w804) -> ("Horizontal"=w801:i32)
                        n671 = for {
                          tunnel: w798 -> [w807] mode=indexing
                          tunnel: [w806] -> w803 mode=indexing
                          n672 = Unbundle By Name(w807) -> ("Vertical"=w806:i32)
                        }
                        n673 = Array Max & Min(array=w803) -> (max value=w799:i32, min value=w800:i32)  [unwired: 2 out]
                      }
                      frame #1 {
                        n674 = Unbundle By Name(w808) -> ("Left"=w813:i16, "Top"=w814:i16, "Right"=w815:i16, "Bottom"=w816:i16)
                        n675 = call "2pparameters.vi"("command"="get") -> ("params out"=w834:T6)  [unwired: 1 in]
                        n676 = call "2pparameters.vi"("command"="get") -> ("params out"=w822:T6)  [unwired: 1 in]
                        n677 = To Double Precision Float(number=w813) -> (double precision float=w849:dbl)
                        n678 = To Double Precision Float(number=w814) -> (double precision float=w817:dbl)
                        n679 = To Double Precision Float(number=w815) -> (double precision float=w850:dbl)
                        n680 = To Double Precision Float(number=w816) -> (double precision float=w818:dbl)
                        n681 = Unbundle By Name(w834) -> ("Vy-max Img"=w836:dbl, "Vy-min Img"=w837:dbl)
                        n682 = Unbundle By Name(w822) -> ("Vx-min Img"=w828:dbl, "VX-max Img"=w823:dbl)
                        n683 = call "2pparameters.vi"("command"="get") -> ("params out"=w827:T6)  [unwired: 1 in]
                        n684 = Subtract(x=w849, y=w850) -> (x-y=w819:dbl)
                        n685 = Subtract(x=w817, y=w818) -> (x-y=w820:dbl)
                        n686 = Subtract(x=w836, y=w837) -> (x-y=w838:dbl)
                        n687 = Subtract(x=w828, y=w823) -> (x-y=w824:dbl)
                        n688 = Unbundle By Name(w827) -> ("Vx-min Img"=w832:dbl, "Vy-max Img"=w840:dbl)
                        n689 = Divide(x=w824, y=w819) -> (x/y=w846:dbl)
                        n690 = Divide(x=w838, y=w820) -> (x/y=w847:dbl)
                        n691 = To Double Precision Float(number=w812) -> (double precision float=w845:dbl)
                        n692 = To Double Precision Float(number=w810) -> (double precision float=w830:dbl)
                        n693 = To Double Precision Float(number=w809) -> (double precision float=w839:dbl)
                        n694 = To Double Precision Float(number=w811) -> (double precision float=w848:dbl)
                        n695 = Multiply(x=w845, y=w846) -> (x*y=w829:dbl)
                        n696 = Multiply(x=w846, y=w830) -> (x*y=w831:dbl)
                        n697 = Multiply(x=w839, y=w847) -> (x*y=w841:dbl)
                        n698 = Multiply(x=w847, y=w848) -> (x*y=w842:dbl)
                        n699 = Add(x=w829, y=w832) -> (x+y=w825:dbl)
                        n700 = Add(x=w831, y=w832) -> (x+y=w833:dbl)
                        n701 = Add(x=w840, y=w841) -> (x+y=w843:dbl)
                        n702 = Add(x=w840, y=w842) -> (x+y=w844:dbl)
                        n703 = local write "Vy-min"(w843) -> ()
                        n704 = local write "Vx-min"(w825) -> ()
                        n705 = local write "Vy-max"(w844) -> ()
                        n706 = local write "Vx-max"(w833) -> ()
                      }
                      frame #2 {
                        n707 = local read "Vy-max"() -> (w876:dbl)
                        n708 = local read "Vy-min"() -> (w877:dbl)
                        n709 = local read "Vx-max"() -> (w874:dbl)
                        n710 = local read "Vx-min"() -> (w875:dbl)
                        n711 = call "2pparameters.vi"("command"="get") -> ("params out"=w864:T6)  [unwired: 1 in]
                        n712 = Unbundle By Name(w864) -> ("VX-max Img"=w866:dbl, "Vx-min Img"=w867:dbl, "Vy-max Img"=w868:dbl, "Vy-min Img"=w869:dbl, "Angle Img"=w859:dbl)
                        n713 = Add(x=w866, y=w867) -> (x+y=w870:dbl)
                        n714 = Add(x=w868, y=w869) -> (x+y=w873:dbl)
                        n715 = Divide(x=w870, y=2.0) -> (x/y=w854:dbl)
                        n716 = Subtract(x=w874, y=w854) -> (x-y=w863:dbl)
                        n717 = Subtract(x=w875, y=w854) -> (x-y=w862:dbl)
                        n718 = Divide(x=w873, y=2.0) -> (x/y=w853:dbl)
                        n719 = Subtract(x=w877, y=w853) -> (x-y=w860:dbl)
                        n720 = Subtract(x=w876, y=w853) -> (x-y=w861:dbl)
                        n721 = script code="Xic=(ximax+ximin)./2;\nYic=(yimax+yimin)./2;\nXicrot=Xic.*cos(pi/180.*phi)+Yic.*sin(pi./180.*phi);\nYicrot=-Xic.*sin(pi./180.*phi)+Yic.*cos(pi./180.*phi);\nxirmax=ximax-Xic+Xicrot;\nxirmin=ximin-Xic+Xicrot;\nyirmax=yimax-Yic+Yicrot;\nyirmin=yimin-Yic+Yicrot;"("ximax"=w863, "ximin"=w862, "yimax"=w861, "yimin"=w860, "phi"=w859) -> ("xirmax"=w858:dbl, "xirmin"=w857:dbl, "yirmax"=w856:dbl, "yirmin"=w855:dbl)  [unwired: 1 in, 1 out]
                        n722 = Add(x=w855, y=w853) -> (x+y=w851:dbl)
                        n723 = Add(x=w856, y=w853) -> (x+y=w852:dbl)
                        n724 = Add(x=w857, y=w854) -> (x+y=w879:dbl)
                        n725 = Add(x=w858, y=w854) -> (x+y=w878:dbl)
                        n726 = local write "Vy-max"(w852) -> ()
                        n727 = local write "Vx-min"(w879) -> ()
                        n728 = local write "Vx-max"(w878) -> ()
                        n729 = local write "Vy-min"(w851) -> ()
                      }
                      frame #3 {
                        n730 = disable-structure shown="Disabled" {
                          disable-tunnel: w881 -> [w893 _]
                          disable-tunnel: w880 -> [w890 _]
                          frame Disabled {
                            n731 = local read "Vx-min"() -> (w888:dbl)
                            n732 = local read "Vx-max"() -> (w889:dbl)
                            n733 = local read "Ypixels"() -> (w891:i32)
                            n734 = local read "Xpixels"() -> (w892:i32)
                            n735 = local read "Vy-max"() -> (w886:dbl)
                            n736 = local read "Vy-min"() -> (w887:dbl)
                            n737 = call "2pparameters.vi"("command"="get") -> ("params out"=w884:T6)  [unwired: 1 in]
                            n738 = Unbundle By Name(w884) -> ("Angle Img"=w883:dbl)
                            n739 = call "ScanningWaveform_v4.vi"("Vy-min"=w887, "Vy-max"=w886, "yPixels/tPixels"=w891, "xPixels/rPixels"=w892, "Vx-min"=w888, "Vx-max"=w889, "Drawing Mode"=w893, "Angle"=w883, "Points"=w890, "points in ellipse"=100.0) -> ()  [unwired: 6 in, 4 out]
                          }
                          frame Enabled {
                          }
                        }
                        n740 = local write "Array"(w880) -> ()
                      }
                    }
                  }
                  frame 4 {
                    n741 = stacked-sequence {
                      seq-local: [w900 _ _ _] -> [_ w954 _ _]
                      seq-local: [w899 _ _ _] -> [_ w953 _ _]
                      seq-local: [w897 _ _ _] -> [_ w952 _ _]
                      seq-local: [w898 _ _ _] -> [_ w951 _ _]
                      tunnel: w896 -> [_ _ _ w991]
                      tunnel: w894 -> [w901 _ _ w988]
                      tunnel: w895 -> [_ w950 _ _]
                      frame #0 {
                        n742 = for {
                          tunnel: w901 -> [w911] mode=indexing
                          shift-right: [w907] -> w899
                          shift-left: 1000 -> [w909]
                          shift-right: [w906] -> w898
                          shift-left: 0 -> [w910]
                          n743 = Unbundle By Name(w911) -> ("Vertical"=w908:i32)
                          n744 = Max & Min(x=w909, y=w908) -> (min(x,y)=w907:i32)  [unwired: 1 out]
                          n745 = Max & Min(x=w908, y=w910) -> (max(x,y)=w906:i32)  [unwired: 1 out]
                        }
                        n746 = Array Max & Min(array=w901) -> (max value=w904:T1, min value=w905:T1)  [unwired: 2 out]
                        n747 = Unbundle By Name(w905) -> ("Horizontal"=w900:i32)
                        n748 = Unbundle By Name(w904) -> ("Horizontal"=w897:i32)
                      }
                      frame #1 {
                        n749 = Unbundle By Name(w950) -> ("Left"=w912:i16, "Top"=w913:i16, "Right"=w914:i16, "Bottom"=w915:i16)
                        n750 = call "2pparameters.vi"("command"="get") -> ("params out"=w933:T6)  [unwired: 1 in]
                        n751 = call "2pparameters.vi"("command"="get") -> ("params out"=w921:T6)  [unwired: 1 in]
                        n752 = To Double Precision Float(number=w912) -> (double precision float=w948:dbl)
                        n753 = To Double Precision Float(number=w913) -> (double precision float=w916:dbl)
                        n754 = To Double Precision Float(number=w914) -> (double precision float=w949:dbl)
                        n755 = To Double Precision Float(number=w915) -> (double precision float=w917:dbl)
                        n756 = Unbundle By Name(w933) -> ("Vy-max Img"=w935:dbl, "Vy-min Img"=w936:dbl)
                        n757 = Unbundle By Name(w921) -> ("Vx-min Img"=w927:dbl, "VX-max Img"=w922:dbl)
                        n758 = call "2pparameters.vi"("command"="get") -> ("params out"=w926:T6)  [unwired: 1 in]
                        n759 = Subtract(x=w948, y=w949) -> (x-y=w918:dbl)
                        n760 = Subtract(x=w916, y=w917) -> (x-y=w919:dbl)
                        n761 = Subtract(x=w935, y=w936) -> (x-y=w937:dbl)
                        n762 = Subtract(x=w927, y=w922) -> (x-y=w923:dbl)
                        n763 = Unbundle By Name(w926) -> ("Vx-min Img"=w931:dbl, "Vy-max Img"=w939:dbl)
                        n764 = Divide(x=w923, y=w918) -> (x/y=w945:dbl)
                        n765 = Divide(x=w937, y=w919) -> (x/y=w946:dbl)
                        n766 = To Double Precision Float(number=w954) -> (double precision float=w944:dbl)
                        n767 = To Double Precision Float(number=w952) -> (double precision float=w929:dbl)
                        n768 = To Double Precision Float(number=w951) -> (double precision float=w938:dbl)
                        n769 = To Double Precision Float(number=w953) -> (double precision float=w947:dbl)
                        n770 = Multiply(x=w944, y=w945) -> (x*y=w928:dbl)
                        n771 = Multiply(x=w945, y=w929) -> (x*y=w930:dbl)
                        n772 = Multiply(x=w938, y=w946) -> (x*y=w940:dbl)
                        n773 = Multiply(x=w946, y=w947) -> (x*y=w941:dbl)
                        n774 = Add(x=w928, y=w931) -> (x+y=w924:dbl)
                        n775 = Add(x=w930, y=w931) -> (x+y=w932:dbl)
                        n776 = Add(x=w939, y=w940) -> (x+y=w942:dbl)
                        n777 = Add(x=w939, y=w941) -> (x+y=w943:dbl)
                        n778 = local write "Vy-min"(w942) -> ()
                        n779 = local write "Vx-min"(w924) -> ()
                        n780 = local write "Vy-max"(w943) -> ()
                        n781 = local write "Vx-max"(w932) -> ()
                      }
                      frame #2 {
                        n782 = local read "Vy-max"() -> (w980:dbl)
                        n783 = local read "Vy-min"() -> (w981:dbl)
                        n784 = local read "Vx-max"() -> (w978:dbl)
                        n785 = local read "Vx-min"() -> (w979:dbl)
                        n786 = call "2pparameters.vi"("command"="get") -> ("params out"=w968:T6)  [unwired: 1 in]
                        n787 = Unbundle By Name(w968) -> ("VX-max Img"=w970:dbl, "Vx-min Img"=w971:dbl, "Vy-max Img"=w972:dbl, "Vy-min Img"=w973:dbl, "Angle Img"=w963:dbl)
                        n788 = Add(x=w970, y=w971) -> (x+y=w974:dbl)
                        n789 = Add(x=w972, y=w973) -> (x+y=w977:dbl)
                        n790 = Divide(x=w974, y=2.0) -> (x/y=w958:dbl)
                        n791 = Subtract(x=w978, y=w958) -> (x-y=w967:dbl)
                        n792 = Subtract(x=w979, y=w958) -> (x-y=w966:dbl)
                        n793 = Divide(x=w977, y=2.0) -> (x/y=w957:dbl)
                        n794 = Subtract(x=w981, y=w957) -> (x-y=w964:dbl)
                        n795 = Subtract(x=w980, y=w957) -> (x-y=w965:dbl)
                        n796 = script code="Xic=(ximax+ximin)./2;\nYic=(yimax+yimin)./2;\nXicrot=Xic.*cos(pi/180.*phi)+Yic.*sin(pi./180.*phi);\nYicrot=-Xic.*sin(pi./180.*phi)+Yic.*cos(pi./180.*phi);\nxirmax=ximax-Xic+Xicrot;\nxirmin=ximin-Xic+Xicrot;\nyirmax=yimax-Yic+Yicrot;\nyirmin=yimin-Yic+Yicrot;"("ximax"=w967, "ximin"=w966, "yimax"=w965, "yimin"=w964, "phi"=w963) -> ("xirmax"=w962:dbl, "xirmin"=w961:dbl, "yirmax"=w960:dbl, "yirmin"=w959:dbl)  [unwired: 1 in, 1 out]
                        n797 = Add(x=w959, y=w957) -> (x+y=w955:dbl)
                        n798 = Add(x=w960, y=w957) -> (x+y=w956:dbl)
                        n799 = Add(x=w961, y=w958) -> (x+y=w983:dbl)
                        n800 = Add(x=w962, y=w958) -> (x+y=w982:dbl)
                        n801 = local write "Vy-max"(w956) -> ()
                        n802 = local write "Vx-min"(w983) -> ()
                        n803 = local write "Vx-max"(w982) -> ()
                        n804 = local write "Vy-min"(w955) -> ()
                      }
                      frame #3 {
                        n805 = local read "Vx-min"() -> (w986:dbl)
                        n806 = local read "Vx-max"() -> (w987:dbl)
                        n807 = local read "Ypixels"() -> (w989:i32)
                        n808 = local read "Xpixels"() -> (w990:i32)
                        n809 = local read "Vy-max"() -> (w984:dbl)
                        n810 = local read "Vy-min"() -> (w985:dbl)
                        n811 = call "ScanningWaveform_v4.vi"("Vy-min"=w985, "Vy-max"=w984, "yPixels/tPixels"=w989, "xPixels/rPixels"=w990, "Vx-min"=w986, "Vx-max"=w987, "Drawing Mode"=w991, "Points"=w988) -> ()  [unwired: 8 in, 4 out]
                        n812 = local write "Array"(w988) -> ()
                      }
                    }
                  }
                  frame 5 {
                    n813 = stacked-sequence {
                      seq-local: [w1006 _ _ _ _ _] -> [_ w1054 _ w1116 _ _]
                      seq-local: [w1003 _ _ _ _ _] -> [_ w1053 _ w1091 _ _]
                      seq-local: [w1005 _ _ _ _ _] -> [_ w1052 _ w1115 _ _]
                      seq-local: [w1004 _ _ _ _ _] -> [_ w1051 _ w1090 _ _]
                      tunnel: w995 -> [w1013 w1048 _ w1113 _ _]
                      tunnel: w994 -> [w1012 _ _ _ _ _]
                      tunnel: w993 -> [w1011 _ _ _ _ _]
                      tunnel: w992 -> [_ _ _ _ _ w1161]
                      frame #0 {
                        w1000 = 2 ("value")
                        n814 = Unbundle By Name(w1011) -> ("Horizontal"=w1017:i32, "Vertical"=w1015:i32)
                        n815 = Unbundle By Name(w1012) -> ("Horizontal"=w1008:i32, "Vertical"=w1007:i32)
                        n816 = Unbundle By Name(w1013) -> ("Left"=w1016:i16, "Top"=w1014:i16)
                        n817 = To Long Integer(number=w1014) -> (32bit integer=w1009:i32)
                        n818 = To Long Integer(number=w1016) -> (32bit integer=w1010:i32)
                        n819 = Compound Arithmetic op=MULTIPLY(w1008, w1000) -> (w1002:i32)
                        n820 = Compound Arithmetic op=MULTIPLY(w1007, w1000) -> (w1001:i32)
                        n821 = Compound Arithmetic op=ADD(invert w1010, w1017) -> (w997:i32)
                        n822 = Compound Arithmetic op=ADD(invert w1009, w1015) -> (w996:i32)
                        n823 = Compound Arithmetic op=ADD(invert w997, w1002) -> (w999:i32)
                        n824 = Compound Arithmetic op=ADD(invert w996, w1001) -> (w998:i32)
                        n825 = Max & Min(x=w997, y=w999) -> (max(x,y)=w1005:i32, min(x,y)=w1006:i32)
                        n826 = Max & Min(x=w996, y=w998) -> (max(x,y)=w1004:i32, min(x,y)=w1003:i32)
                      }
                      frame #1 {
                        n827 = Unbundle By Name(w1048) -> ("Left"=w1060:i16, "Top"=w1059:i16, "Right"=w1058:i16, "Bottom"=w1057:i16)
                        n828 = call "2pparameters.vi"("command"="get") -> ("params out"=w1046:T6)  [unwired: 1 in]
                        n829 = call "2pparameters.vi"("command"="get") -> ("params out"=w1034:T6)  [unwired: 1 in]
                        n830 = To Double Precision Float(number=w1060) -> (double precision float=w1019:dbl)
                        n831 = To Double Precision Float(number=w1059) -> (double precision float=w1056:dbl)
                        n832 = To Double Precision Float(number=w1058) -> (double precision float=w1018:dbl)
                        n833 = To Double Precision Float(number=w1057) -> (double precision float=w1055:dbl)
                        n834 = Unbundle By Name(w1046) -> ("Vx-min Img"=w1040:dbl, "VX-max Img"=w1045:dbl)
                        n835 = Unbundle By Name(w1034) -> ("Vy-max Img"=w1032:dbl, "Vy-min Img"=w1031:dbl)
                        n836 = call "2pparameters.vi"("command"="get") -> ("params out"=w1041:T6)  [unwired: 1 in]
                        n837 = Subtract(x=w1040, y=w1045) -> (x-y=w1044:dbl)
                        n838 = Subtract(x=w1019, y=w1018) -> (x-y=w1050:dbl)
                        n839 = Subtract(x=w1056, y=w1055) -> (x-y=w1049:dbl)
                        n840 = Subtract(x=w1032, y=w1031) -> (x-y=w1030:dbl)
                        n841 = Unbundle By Name(w1041) -> ("Vx-min Img"=w1036:dbl, "Vy-max Img"=w1028:dbl)
                        n842 = Divide(x=w1044, y=w1050) -> (x/y=w1022:dbl)
                        n843 = Divide(x=w1030, y=w1049) -> (x/y=w1021:dbl)
                        n844 = To Double Precision Float(number=w1054) -> (double precision float=w1023:dbl)
                        n845 = To Double Precision Float(number=w1052) -> (double precision float=w1038:dbl)
                        n846 = To Double Precision Float(number=w1051) -> (double precision float=w1029:dbl)
                        n847 = To Double Precision Float(number=w1053) -> (double precision float=w1020:dbl)
                        n848 = Multiply(x=w1023, y=w1022) -> (x*y=w1039:dbl)
                        n849 = Multiply(x=w1022, y=w1038) -> (x*y=w1037:dbl)
                        n850 = Multiply(x=w1029, y=w1021) -> (x*y=w1027:dbl)
                        n851 = Multiply(x=w1021, y=w1020) -> (x*y=w1026:dbl)
                        n852 = Add(x=w1039, y=w1036) -> (x+y=w1043:dbl)
                        n853 = Add(x=w1037, y=w1036) -> (x+y=w1035:dbl)
                        n854 = Add(x=w1028, y=w1027) -> (x+y=w1025:dbl)
                        n855 = Add(x=w1028, y=w1026) -> (x+y=w1024:dbl)
                        n856 = local write "Vy-min"(w1025) -> ()
                        n857 = local write "Vx-min"(w1043) -> ()
                        n858 = local write "Vy-max"(w1024) -> ()
                        n859 = local write "Vx-max"(w1035) -> ()
                      }
                      frame #2 {
                        n860 = local read "Vy-max"() -> (w1086:dbl)
                        n861 = local read "Vy-min"() -> (w1087:dbl)
                        n862 = local read "Vx-max"() -> (w1084:dbl)
                        n863 = local read "Vx-min"() -> (w1085:dbl)
                        n864 = call "2pparameters.vi"("command"="get") -> ("params out"=w1074:T6)  [unwired: 1 in]
                        n865 = Unbundle By Name(w1074) -> ("VX-max Img"=w1076:dbl, "Vx-min Img"=w1077:dbl, "Vy-max Img"=w1078:dbl, "Vy-min Img"=w1079:dbl, "Angle Img"=w1069:dbl)
                        n866 = Add(x=w1076, y=w1077) -> (x+y=w1080:dbl)
                        n867 = Add(x=w1078, y=w1079) -> (x+y=w1083:dbl)
                        n868 = Divide(x=w1080, y=2.0) -> (x/y=w1064:dbl)
                        n869 = Subtract(x=w1084, y=w1064) -> (x-y=w1073:dbl)
                        n870 = Subtract(x=w1085, y=w1064) -> (x-y=w1072:dbl)
                        n871 = Divide(x=w1083, y=2.0) -> (x/y=w1063:dbl)
                        n872 = Subtract(x=w1087, y=w1063) -> (x-y=w1070:dbl)
                        n873 = Subtract(x=w1086, y=w1063) -> (x-y=w1071:dbl)
                        n874 = script code="Xic=(ximax+ximin)./2;\nYic=(yimax+yimin)./2;\nXicrot=Xic.*cos(pi/180.*phi)+Yic.*sin(pi./180.*phi);\nYicrot=-Xic.*sin(pi./180.*phi)+Yic.*cos(pi./180.*phi);\nxirmax=ximax-Xic+Xicrot;\nxirmin=ximin-Xic+Xicrot;\nyirmax=yimax-Yic+Yicrot;\nyirmin=yimin-Yic+Yicrot;"("ximax"=w1073, "ximin"=w1072, "yimax"=w1071, "yimin"=w1070, "phi"=w1069) -> ("xirmax"=w1068:dbl, "xirmin"=w1067:dbl, "yirmax"=w1066:dbl, "yirmin"=w1065:dbl)  [unwired: 1 in, 1 out]
                        n875 = Add(x=w1065, y=w1063) -> (x+y=w1061:dbl)
                        n876 = Add(x=w1066, y=w1063) -> (x+y=w1062:dbl)
                        n877 = Add(x=w1067, y=w1064) -> (x+y=w1089:dbl)
                        n878 = Add(x=w1068, y=w1064) -> (x+y=w1088:dbl)
                        n879 = local write "Vy-max"(w1062) -> ()
                        n880 = local write "Vx-min"(w1089) -> ()
                        n881 = local write "Vx-max"(w1088) -> ()
                        n882 = local write "Vy-min"(w1061) -> ()
                      }
                      frame #3 {
                        n883 = Unbundle By Name(w1113) -> ("Left"=w1122:i16, "Top"=w1121:i16, "Right"=w1120:i16, "Bottom"=w1119:i16)
                        n884 = To Double Precision Float(number=w1122) -> (double precision float=w1107:dbl)
                        n885 = To Double Precision Float(number=w1121) -> (double precision float=w1118:dbl)
                        n886 = To Double Precision Float(number=w1120) -> (double precision float=w1106:dbl)
                        n887 = To Double Precision Float(number=w1119) -> (double precision float=w1117:dbl)
                        n888 = call "2pparameters.vi"("command"="get") -> ("params out"=w1112:T6)  [unwired: 1 in]
                        n889 = Subtract(x=w1107, y=w1106) -> (x-y=w1114:dbl)
                        n890 = Subtract(x=w1118, y=w1117) -> (x-y=w1092:dbl)
                        n891 = Unbundle By Name(w1112) -> ("Xpixels Img"=w1104:i32, "Ypixels Img"=w1103:i32)
                        n892 = To Double Precision Float(number=w1116) -> (double precision float=w1110:dbl)
                        n893 = To Double Precision Float(number=w1115) -> (double precision float=w1105:dbl)
                        n894 = To Double Precision Float(number=w1091) -> (double precision float=w1109:dbl)
                        n895 = To Double Precision Float(number=w1090) -> (double precision float=w1108:dbl)
                        n896 = To Double Precision Float(number=w1104) -> (double precision float=w1100:dbl)
                        n897 = To Double Precision Float(number=w1103) -> (double precision float=w1098:dbl)
                        n898 = Subtract(x=w1109, y=w1108) -> (x-y=w1099:dbl)
                        n899 = Subtract(x=w1110, y=w1105) -> (x-y=w1102:dbl)
                        n900 = Divide(x=w1102, y=w1114) -> (x/y=w1101:dbl)
                        n901 = Divide(x=w1099, y=w1092) -> (x/y=w1097:dbl)
                        n902 = Multiply(x=w1101, y=w1100) -> (x*y=w1095:dbl)
                        n903 = Multiply(x=w1098, y=w1097) -> (x*y=w1096:dbl)
                        n904 = To Long Integer(number=w1095) -> (32bit integer=w1094:i32)
                        n905 = To Long Integer(number=w1096) -> (32bit integer=w1093:i32)
                        n906 = local write "Xpixels"(w1094) -> ()
                        n907 = local write "Ypixels"(w1093) -> ()
                      }
                      frame #4 {
                        n908 = local read "square pixels"() -> (w1123:bool)
                        n909 = case shown="True" w1123 {
                          frame False {
                            n910 = local read "square matrix"() -> (w1124:bool)
                            n911 = case shown="True" w1124 {
                              frame False {
                              }
                              frame True {
                                n912 = local read "Xpixels"() -> (w1127:i32)
                                n913 = local read "Ypixels"() -> (w1126:i32)
                                n914 = Max & Min(x=w1127, y=w1126) -> (max(x,y)=w1125:i32)  [unwired: 1 out]
                                n915 = local write "Ypixels"(w1125) -> ()
                                n916 = local write "Xpixels"(w1125) -> ()
                              }
                            }
                          }
                          frame True {
                            n917 = local read "square matrix"() -> (w1128:bool)
                            n918 = case shown="False" w1128 {
                              frame False {
                                n919 = local read "Vy-min"() -> (w1138:dbl)
                                n920 = local read "Vx-max"() -> (w1142:dbl)
                                n921 = local read "Vx-min"() -> (w1141:dbl)
                                n922 = local read "Vy-max"() -> (w1137:dbl)
                                n923 = Subtract(x=w1137, y=w1138) -> (x-y=w1139:dbl)
                                n924 = Subtract(x=w1142, y=w1141) -> (x-y=w1140:dbl)
                                n925 = Absolute Value(x=w1139) -> (abs(x)=w1130:dbl)
                                n926 = Absolute Value(x=w1140) -> (abs(x)=w1131:dbl)
                                n927 = local read "Xpixels"() -> (w1135:i32)
                                n928 = Divide(x=w1131, y=w1130) -> (x/y=w1136:dbl)
                                n929 = local read "Ypixels"() -> (w1132:i32)
                                n930 = Greater Or Equal?(x=w1131, y=w1130) -> (x >= y?=w1129:bool)
                                n931 = case shown="False" w1129 {
                                tunnel: w1136 -> [w1147 w1150]
                                tunnel: w1135 -> [w1144 _]
                                tunnel: [w1144 w1149] -> w1134
                                tunnel: [w1143 w1148] -> w1133
                                tunnel: w1132 -> [_ w1148]
                                frame False {
                                n932 = To Double Precision Float(number=w1144) -> (double precision float=w1146:dbl)
                                n933 = Divide(x=w1146, y=w1147) -> (x/y=w1145:dbl)
                                n934 = To Long Integer(number=w1145) -> (32bit integer=w1143:i32)
                                }
                                frame True {
                                n935 = To Double Precision Float(number=w1148) -> (double precision float=w1152:dbl)
                                n936 = Multiply(x=w1152, y=w1150) -> (x*y=w1151:dbl)
                                n937 = To Long Integer(number=w1151) -> (32bit integer=w1149:i32)
                                }
                                }
                                n938 = local write "Xpixels"(w1134) -> ()
                                n939 = local write "Ypixels"(w1133) -> ()
                              }
                              frame True {
                              }
                            }
                          }
                        }
                      }
                      frame #5 {
                        n940 = local read "Vy-min"() -> (w1154:dbl)
                        n941 = local read "Vx-max"() -> (w1157:dbl)
                        n942 = local read "Vx-min"() -> (w1156:dbl)
                        n943 = local read "Vy-max"() -> (w1155:dbl)
                        n944 = local read "Ypixels"() -> (w1159:i32)
                        n945 = local read "Xpixels"() -> (w1160:i32)
                        n946 = local read "Angle"() -> (w1158:dbl)
                        n947 = call "ScanningWaveform_v4.vi"("Vy-min"=w1154, "Vy-max"=w1155, "yPixels/tPixels"=w1159, "xPixels/rPixels"=w1160, "Vx-min"=w1156, "Vx-max"=w1157, "Drawing Mode"=w1161, "Angle"=w1158, "points in ellipse"=100.0) -> ()  [unwired: 7 in, 4 out]
                      }
                    }
                  }
                  frame 6 {
                    n948 = stacked-sequence {
                      seq-local: [w1169 _ _ _ _ _] -> [_ w1221 _ w1283 _ _]
                      seq-local: [w1166 _ _ _ _ _] -> [_ w1220 _ w1258 _ _]
                      seq-local: [w1168 _ _ _ _ _] -> [_ w1219 _ w1282 _ _]
                      seq-local: [w1167 _ _ _ _ _] -> [_ w1218 _ w1257 _ _]
                      tunnel: w1165 -> [w1178 w1215 _ w1280 _ _]
                      tunnel: w1164 -> [w1177 _ _ _ _ _]
                      tunnel: w1163 -> [w1176 _ _ _ _ _]
                      tunnel: w1162 -> [_ _ _ _ _ w1327]
                      frame #0 {
                        n949 = Unbundle By Name(w1176) -> ("Horizontal"=w1184:i32, "Vertical"=w1181:i32)
                        n950 = Unbundle By Name(w1177) -> ("Horizontal"=w1173:i32, "Vertical"=w1172:i32)
                        n951 = Unbundle By Name(w1178) -> ("Left"=w1182:i16, "Top"=w1179:i16, "Right"=w1171:i16, "Bottom"=w1170:i16)
                        n952 = To Long Integer(number=w1179) -> (32bit integer=w1174:i32)
                        n953 = To Long Integer(number=w1182) -> (32bit integer=w1175:i32)
                        n954 = To Long Integer(number=w1170) -> ()  [unwired: 1 out]
                        n955 = To Long Integer(number=w1171) -> ()  [unwired: 1 out]
                        n956 = Compound Arithmetic op=ADD(invert w1175, w1184) -> (w1183:i32)
                        n957 = Compound Arithmetic op=ADD(invert w1174, w1181) -> (w1180:i32)
                        n958 = Max & Min(x=w1183, y=w1173) -> (max(x,y)=w1168:i32, min(x,y)=w1169:i32)
                        n959 = Max & Min(x=w1180, y=w1172) -> (max(x,y)=w1167:i32, min(x,y)=w1166:i32)
                      }
                      frame #1 {
                        n960 = Unbundle By Name(w1215) -> ("Left"=w1227:i16, "Top"=w1226:i16, "Right"=w1225:i16, "Bottom"=w1224:i16)
                        n961 = call "2pparameters.vi"("command"="get") -> ("params out"=w1213:T6)  [unwired: 1 in]
                        n962 = call "2pparameters.vi"("command"="get") -> ("params out"=w1201:T6)  [unwired: 1 in]
                        n963 = To Double Precision Float(number=w1227) -> (double precision float=w1186:dbl)
                        n964 = To Double Precision Float(number=w1226) -> (double precision float=w1223:dbl)
                        n965 = To Double Precision Float(number=w1225) -> (double precision float=w1185:dbl)
                        n966 = To Double Precision Float(number=w1224) -> (double precision float=w1222:dbl)
                        n967 = Unbundle By Name(w1213) -> ("Vx-min Img"=w1207:dbl, "VX-max Img"=w1212:dbl)
                        n968 = Unbundle By Name(w1201) -> ("Vy-max Img"=w1199:dbl, "Vy-min Img"=w1198:dbl)
                        n969 = call "2pparameters.vi"("command"="get") -> ("params out"=w1208:T6)  [unwired: 1 in]
                        n970 = Subtract(x=w1207, y=w1212) -> (x-y=w1211:dbl)
                        n971 = Subtract(x=w1186, y=w1185) -> (x-y=w1217:dbl)
                        n972 = Subtract(x=w1223, y=w1222) -> (x-y=w1216:dbl)
                        n973 = Subtract(x=w1199, y=w1198) -> (x-y=w1197:dbl)
                        n974 = Unbundle By Name(w1208) -> ("Vx-min Img"=w1203:dbl, "Vy-max Img"=w1195:dbl)
                        n975 = Divide(x=w1211, y=w1217) -> (x/y=w1189:dbl)
                        n976 = Divide(x=w1197, y=w1216) -> (x/y=w1188:dbl)
                        n977 = To Double Precision Float(number=w1221) -> (double precision float=w1190:dbl)
                        n978 = To Double Precision Float(number=w1219) -> (double precision float=w1205:dbl)
                        n979 = To Double Precision Float(number=w1218) -> (double precision float=w1196:dbl)
                        n980 = To Double Precision Float(number=w1220) -> (double precision float=w1187:dbl)
                        n981 = Multiply(x=w1190, y=w1189) -> (x*y=w1206:dbl)
                        n982 = Multiply(x=w1189, y=w1205) -> (x*y=w1204:dbl)
                        n983 = Multiply(x=w1196, y=w1188) -> (x*y=w1194:dbl)
                        n984 = Multiply(x=w1188, y=w1187) -> (x*y=w1193:dbl)
                        n985 = Add(x=w1206, y=w1203) -> (x+y=w1210:dbl)
                        n986 = Add(x=w1204, y=w1203) -> (x+y=w1202:dbl)
                        n987 = Add(x=w1195, y=w1194) -> (x+y=w1192:dbl)
                        n988 = Add(x=w1195, y=w1193) -> (x+y=w1191:dbl)
                        n989 = local write "Vy-min"(w1192) -> ()
                        n990 = local write "Vx-min"(w1210) -> ()
                        n991 = local write "Vy-max"(w1191) -> ()
                        n992 = local write "Vx-max"(w1202) -> ()
                      }
                      frame #2 {
                        n993 = local read "Vy-max"() -> (w1253:dbl)
                        n994 = local read "Vy-min"() -> (w1254:dbl)
                        n995 = local read "Vx-max"() -> (w1251:dbl)
                        n996 = local read "Vx-min"() -> (w1252:dbl)
                        n997 = call "2pparameters.vi"("command"="get") -> ("params out"=w1241:T6)  [unwired: 1 in]
                        n998 = Unbundle By Name(w1241) -> ("VX-max Img"=w1243:dbl, "Vx-min Img"=w1244:dbl, "Vy-max Img"=w1245:dbl, "Vy-min Img"=w1246:dbl, "Angle Img"=w1236:dbl)
                        n999 = Add(x=w1243, y=w1244) -> (x+y=w1247:dbl)
                        n1000 = Add(x=w1245, y=w1246) -> (x+y=w1250:dbl)
                        n1001 = Divide(x=w1247, y=2.0) -> (x/y=w1231:dbl)
                        n1002 = Subtract(x=w1251, y=w1231) -> (x-y=w1240:dbl)
                        n1003 = Subtract(x=w1252, y=w1231) -> (x-y=w1239:dbl)
                        n1004 = Divide(x=w1250, y=2.0) -> (x/y=w1230:dbl)
                        n1005 = Subtract(x=w1254, y=w1230) -> (x-y=w1237:dbl)
                        n1006 = Subtract(x=w1253, y=w1230) -> (x-y=w1238:dbl)
                        n1007 = script code="Xic=(ximax+ximin)./2;\nYic=(yimax+yimin)./2;\nXicrot=Xic.*cos(pi/180.*phi)+Yic.*sin(pi./180.*phi);\nYicrot=-Xic.*sin(pi./180.*phi)+Yic.*cos(pi./180.*phi);\nxirmax=ximax-Xic+Xicrot;\nxirmin=ximin-Xic+Xicrot;\nyirmax=yimax-Yic+Yicrot;\nyirmin=yimin-Yic+Yicrot;"("ximax"=w1240, "ximin"=w1239, "yimax"=w1238, "yimin"=w1237, "phi"=w1236) -> ("xirmax"=w1235:dbl, "xirmin"=w1234:dbl, "yirmax"=w1233:dbl, "yirmin"=w1232:dbl)  [unwired: 1 in, 1 out]
                        n1008 = Add(x=w1232, y=w1230) -> (x+y=w1228:dbl)
                        n1009 = Add(x=w1233, y=w1230) -> (x+y=w1229:dbl)
                        n1010 = Add(x=w1234, y=w1231) -> (x+y=w1256:dbl)
                        n1011 = Add(x=w1235, y=w1231) -> (x+y=w1255:dbl)
                        n1012 = local write "Vy-max"(w1229) -> ()
                        n1013 = local write "Vx-min"(w1256) -> ()
                        n1014 = local write "Vx-max"(w1255) -> ()
                        n1015 = local write "Vy-min"(w1228) -> ()
                      }
                      frame #3 {
                        n1016 = Unbundle By Name(w1280) -> ("Left"=w1289:i16, "Top"=w1288:i16, "Right"=w1287:i16, "Bottom"=w1286:i16)
                        n1017 = To Double Precision Float(number=w1289) -> (double precision float=w1274:dbl)
                        n1018 = To Double Precision Float(number=w1288) -> (double precision float=w1285:dbl)
                        n1019 = To Double Precision Float(number=w1287) -> (double precision float=w1273:dbl)
                        n1020 = To Double Precision Float(number=w1286) -> (double precision float=w1284:dbl)
                        n1021 = call "2pparameters.vi"("command"="get") -> ("params out"=w1279:T6)  [unwired: 1 in]
                        n1022 = Subtract(x=w1274, y=w1273) -> (x-y=w1281:dbl)
                        n1023 = Subtract(x=w1285, y=w1284) -> (x-y=w1259:dbl)
                        n1024 = Unbundle By Name(w1279) -> ("Xpixels Img"=w1271:i32, "Ypixels Img"=w1270:i32)
                        n1025 = To Double Precision Float(number=w1283) -> (double precision float=w1277:dbl)
                        n1026 = To Double Precision Float(number=w1282) -> (double precision float=w1272:dbl)
                        n1027 = To Double Precision Float(number=w1258) -> (double precision float=w1276:dbl)
                        n1028 = To Double Precision Float(number=w1257) -> (double precision float=w1275:dbl)
                        n1029 = To Double Precision Float(number=w1271) -> (double precision float=w1267:dbl)
                        n1030 = To Double Precision Float(number=w1270) -> (double precision float=w1265:dbl)
                        n1031 = Subtract(x=w1276, y=w1275) -> (x-y=w1266:dbl)
                        n1032 = Subtract(x=w1277, y=w1272) -> (x-y=w1269:dbl)
                        n1033 = Divide(x=w1269, y=w1281) -> (x/y=w1268:dbl)
                        n1034 = Divide(x=w1266, y=w1259) -> (x/y=w1264:dbl)
                        n1035 = Multiply(x=w1268, y=w1267) -> (x*y=w1262:dbl)
                        n1036 = Multiply(x=w1265, y=w1264) -> (x*y=w1263:dbl)
                        n1037 = To Long Integer(number=w1262) -> (32bit integer=w1261:i32)
                        n1038 = To Long Integer(number=w1263) -> (32bit integer=w1260:i32)
                        n1039 = local write "Xpixels"(w1261) -> ()
                        n1040 = local write "Ypixels"(w1260) -> ()
                      }
                      frame #4 {
                        n1041 = local read "square pixels"() -> (w1290:bool)
                        n1042 = case shown="True" w1290 {
                          frame False {
                            n1043 = local read "square matrix"() -> (w1291:bool)
                            n1044 = case shown="True" w1291 {
                              frame False {
                              }
                              frame True {
                                n1045 = local read "Xpixels"() -> (w1294:i32)
                                n1046 = local read "Ypixels"() -> (w1293:i32)
                                n1047 = Max & Min(x=w1294, y=w1293) -> (max(x,y)=w1292:i32)  [unwired: 1 out]
                                n1048 = local write "Ypixels"(w1292) -> ()
                                n1049 = local write "Xpixels"(w1292) -> ()
                              }
                            }
                          }
                          frame True {
                            n1050 = local read "square matrix"() -> (w1295:bool)
                            n1051 = case shown="False" w1295 {
                              frame False {
                                n1052 = local read "Vy-min"() -> (w1305:dbl)
                                n1053 = local read "Vx-max"() -> (w1309:dbl)
                                n1054 = local read "Vx-min"() -> (w1308:dbl)
                                n1055 = local read "Vy-max"() -> (w1304:dbl)
                                n1056 = Subtract(x=w1304, y=w1305) -> (x-y=w1306:dbl)
                                n1057 = Subtract(x=w1309, y=w1308) -> (x-y=w1307:dbl)
                                n1058 = Absolute Value(x=w1306) -> (abs(x)=w1297:dbl)
                                n1059 = Absolute Value(x=w1307) -> (abs(x)=w1298:dbl)
                                n1060 = local read "Xpixels"() -> (w1302:i32)
                                n1061 = Divide(x=w1298, y=w1297) -> (x/y=w1303:dbl)
                                n1062 = local read "Ypixels"() -> (w1299:i32)
                                n1063 = Greater Or Equal?(x=w1298, y=w1297) -> (x >= y?=w1296:bool)
                                n1064 = case shown="False" w1296 {
                                tunnel: w1303 -> [w1314 w1317]
                                tunnel: w1302 -> [w1311 _]
                                tunnel: [w1311 w1316] -> w1301
                                tunnel: [w1310 w1315] -> w1300
                                tunnel: w1299 -> [_ w1315]
                                frame False {
                                n1065 = To Double Precision Float(number=w1311) -> (double precision float=w1313:dbl)
                                n1066 = Divide(x=w1313, y=w1314) -> (x/y=w1312:dbl)
                                n1067 = To Long Integer(number=w1312) -> (32bit integer=w1310:i32)
                                }
                                frame True {
                                n1068 = To Double Precision Float(number=w1315) -> (double precision float=w1319:dbl)
                                n1069 = Multiply(x=w1319, y=w1317) -> (x*y=w1318:dbl)
                                n1070 = To Long Integer(number=w1318) -> (32bit integer=w1316:i32)
                                }
                                }
                                n1071 = local write "Xpixels"(w1301) -> ()
                                n1072 = local write "Ypixels"(w1300) -> ()
                              }
                              frame True {
                              }
                            }
                          }
                        }
                      }
                      frame #5 {
                        n1073 = local read "Vy-min"() -> (w1320:dbl)
                        n1074 = local read "Vx-max"() -> (w1323:dbl)
                        n1075 = local read "Vx-min"() -> (w1322:dbl)
                        n1076 = local read "Vy-max"() -> (w1321:dbl)
                        n1077 = local read "Ypixels"() -> (w1325:i32)
                        n1078 = local read "Xpixels"() -> (w1326:i32)
                        n1079 = local read "Angle"() -> (w1324:dbl)
                        n1080 = call "ScanningWaveform_v4.vi"("Vy-min"=w1320, "Vy-max"=w1321, "yPixels/tPixels"=w1325, "xPixels/rPixels"=w1326, "Vx-min"=w1322, "Vx-max"=w1323, "Drawing Mode"=w1327, "Angle"=w1324) -> ()  [unwired: 8 in, 4 out]
                      }
                    }
                  }
                }
              }
              frame True {
                w1330 = 360.0
                n1081 = Compound Arithmetic op=MULTIPLY(w1328, invert 6.283185307179586, w1330) -> (w1331:dbl)
                n1082 = Quotient & Remainder(x=w1331, y=w1330) -> (x-y*floor(x/y)=w1329:dbl)  [unwired: 1 out]
                n1083 = local write "Angle"(w1329) -> ()
              }
            }
          }
          event "Colormap": Value Change {
            n1084 = event-data() -> ()  [unwired: 1 in, 1 out]
            n1085 = call "misc-global.vi"("command"="get") -> ("misc out"=w1336:cluster{"Colormaps":u32[][]})  [unwired: 1 in]
            n1086 = Unbundle By Name(w1336) -> ("Colormaps"=w1337:u32[][])
            n1087 = Index Array(array=w1337, index (row)="Colormap") -> (element=w1338:u32[])  [unwired: 1 in]
            n1088 = control-ref of="Image"() -> (w1334:refnum<vi>)
            n1089 = property class="IntGraph (strict)"(reference=w1334, "Color Table"=w1338) -> ()  [unwired: 1 in, 2 out]
          }
          event "square pixels": Value Change {
            n1090 = event-data() -> ()  [unwired: 1 in, 1 out]
            n1091 = case shown="True" "square pixels" {
              frame False {
              }
              frame True {
                n1092 = stacked-sequence {
                  frame #0 {
                    n1093 = property on="square pixels" class="Bool (strict)"("Value"=TRUE ("square matrix")) -> ()  [unwired: 2 in, 2 out]
                    n1094 = property on="square matrix" class="Bool (strict)"("Value"=FALSE ("square matrix")) -> ()  [unwired: 2 in, 2 out]
                  }
                  frame #1 {
                    n1095 = local read "square pixels"() -> (w1342:bool)
                    n1096 = case shown="True" w1342 {
                      frame False {
                        n1097 = local read "square matrix"() -> (w1343:bool)
                        n1098 = case shown="True" w1343 {
                          frame False {
                          }
                          frame True {
                            n1099 = local read "Xpixels"() -> (w1346:i32)
                            n1100 = local read "Ypixels"() -> (w1345:i32)
                            n1101 = Max & Min(x=w1346, y=w1345) -> (max(x,y)=w1344:i32)  [unwired: 1 out]
                            n1102 = local write "Ypixels"(w1344) -> ()
                            n1103 = local write "Xpixels"(w1344) -> ()
                          }
                        }
                      }
                      frame True {
                        n1104 = local read "square matrix"() -> (w1347:bool)
                        n1105 = case shown="False" w1347 {
                          frame False {
                            n1106 = local read "Vy-min"() -> (w1357:dbl)
                            n1107 = local read "Vx-max"() -> (w1361:dbl)
                            n1108 = local read "Vx-min"() -> (w1360:dbl)
                            n1109 = local read "Vy-max"() -> (w1356:dbl)
                            n1110 = Subtract(x=w1356, y=w1357) -> (x-y=w1358:dbl)
                            n1111 = Subtract(x=w1361, y=w1360) -> (x-y=w1359:dbl)
                            n1112 = Absolute Value(x=w1358) -> (abs(x)=w1349:dbl)
                            n1113 = Absolute Value(x=w1359) -> (abs(x)=w1350:dbl)
                            n1114 = local read "Xpixels"() -> (w1354:i32)
                            n1115 = Divide(x=w1350, y=w1349) -> (x/y=w1355:dbl)
                            n1116 = local read "Ypixels"() -> (w1351:i32)
                            n1117 = Greater Or Equal?(x=w1350, y=w1349) -> (x >= y?=w1348:bool)
                            n1118 = case shown="False" w1348 {
                              tunnel: w1355 -> [w1366 w1369]
                              tunnel: w1354 -> [w1363 _]
                              tunnel: [w1363 w1368] -> w1353
                              tunnel: [w1362 w1367] -> w1352
                              tunnel: w1351 -> [_ w1367]
                              frame False {
                                n1119 = To Double Precision Float(number=w1363) -> (double precision float=w1365:dbl)
                                n1120 = Divide(x=w1365, y=w1366) -> (x/y=w1364:dbl)
                                n1121 = To Long Integer(number=w1364) -> (32bit integer=w1362:i32)
                              }
                              frame True {
                                n1122 = To Double Precision Float(number=w1367) -> (double precision float=w1371:dbl)
                                n1123 = Multiply(x=w1371, y=w1369) -> (x*y=w1370:dbl)
                                n1124 = To Long Integer(number=w1370) -> (32bit integer=w1368:i32)
                              }
                            }
                            n1125 = local write "Xpixels"(w1353) -> ()
                            n1126 = local write "Ypixels"(w1352) -> ()
                          }
                          frame True {
                          }
                        }
                      }
                    }
                  }
                }
              }
            }
          }
          event "square matrix": Value Change {
            n1127 = event-data() -> ()  [unwired: 1 in, 1 out]
            n1128 = case shown="True" "square matrix" {
              frame False {
              }
              frame True {
                n1129 = stacked-sequence {
                  frame #0 {
                    n1130 = property on="square matrix" class="Bool (strict)"("Value"=TRUE ("square matrix")) -> ()  [unwired: 2 in, 2 out]
                    n1131 = property on="square pixels" class="Bool (strict)"("Value"=FALSE ("square matrix")) -> ()  [unwired: 2 in, 2 out]
                  }
                  frame #1 {
                    n1132 = local read "square pixels"() -> (w1375:bool)
                    n1133 = case shown="True" w1375 {
                      frame False {
                        n1134 = local read "square matrix"() -> (w1376:bool)
                        n1135 = case shown="True" w1376 {
                          frame False {
                          }
                          frame True {
                            n1136 = local read "Xpixels"() -> (w1379:i32)
                            n1137 = local read "Ypixels"() -> (w1378:i32)
                            n1138 = Max & Min(x=w1379, y=w1378) -> (max(x,y)=w1377:i32)  [unwired: 1 out]
                            n1139 = local write "Ypixels"(w1377) -> ()
                            n1140 = local write "Xpixels"(w1377) -> ()
                          }
                        }
                      }
                      frame True {
                        n1141 = local read "square matrix"() -> (w1380:bool)
                        n1142 = case shown="False" w1380 {
                          frame False {
                            n1143 = local read "Vy-min"() -> (w1390:dbl)
                            n1144 = local read "Vx-max"() -> (w1394:dbl)
                            n1145 = local read "Vx-min"() -> (w1393:dbl)
                            n1146 = local read "Vy-max"() -> (w1389:dbl)
                            n1147 = Subtract(x=w1389, y=w1390) -> (x-y=w1391:dbl)
                            n1148 = Subtract(x=w1394, y=w1393) -> (x-y=w1392:dbl)
                            n1149 = Absolute Value(x=w1391) -> (abs(x)=w1382:dbl)
                            n1150 = Absolute Value(x=w1392) -> (abs(x)=w1383:dbl)
                            n1151 = local read "Xpixels"() -> (w1387:i32)
                            n1152 = Divide(x=w1383, y=w1382) -> (x/y=w1388:dbl)
                            n1153 = local read "Ypixels"() -> (w1384:i32)
                            n1154 = Greater Or Equal?(x=w1383, y=w1382) -> (x >= y?=w1381:bool)
                            n1155 = case shown="False" w1381 {
                              tunnel: w1388 -> [w1399 w1402]
                              tunnel: w1387 -> [w1396 _]
                              tunnel: [w1396 w1401] -> w1386
                              tunnel: [w1395 w1400] -> w1385
                              tunnel: w1384 -> [_ w1400]
                              frame False {
                                n1156 = To Double Precision Float(number=w1396) -> (double precision float=w1398:dbl)
                                n1157 = Divide(x=w1398, y=w1399) -> (x/y=w1397:dbl)
                                n1158 = To Long Integer(number=w1397) -> (32bit integer=w1395:i32)
                              }
                              frame True {
                                n1159 = To Double Precision Float(number=w1400) -> (double precision float=w1404:dbl)
                                n1160 = Multiply(x=w1404, y=w1402) -> (x*y=w1403:dbl)
                                n1161 = To Long Integer(number=w1403) -> (32bit integer=w1401:i32)
                              }
                            }
                            n1162 = local write "Xpixels"(w1386) -> ()
                            n1163 = local write "Ypixels"(w1385) -> ()
                          }
                          frame True {
                          }
                        }
                      }
                    }
                  }
                }
              }
            }
          }
          event "Xpixels": Value Change {
            n1164 = event-data() -> ()  [unwired: 1 in, 1 out]
            n1165 = local read "square pixels"() -> (w1405:bool)
            n1166 = case shown="True" w1405 {
              frame False {
                n1167 = local read "square matrix"() -> (w1406:bool)
                n1168 = case shown="True" w1406 {
                  frame False {
                  }
                  frame True {
                    n1169 = local read "Xpixels"() -> (w1407:i32)
                    n1170 = local write "Ypixels"(w1407) -> ()
                    n1171 = local write "Xpixels"(w1407) -> ()
                  }
                }
              }
              frame True {
                n1172 = local read "square matrix"() -> (w1408:bool)
                n1173 = case shown="False" w1408 {
                  frame False {
                    n1174 = local read "Vy-min"() -> (w1417:dbl)
                    n1175 = local read "Vx-max"() -> (w1421:dbl)
                    n1176 = local read "Vx-min"() -> (w1420:dbl)
                    n1177 = local read "Vy-max"() -> (w1416:dbl)
                    n1178 = Subtract(x=w1416, y=w1417) -> (x-y=w1418:dbl)
                    n1179 = Subtract(x=w1421, y=w1420) -> (x-y=w1419:dbl)
                    n1180 = Absolute Value(x=w1418) -> (abs(x)=w1411:dbl)
                    n1181 = Absolute Value(x=w1419) -> (abs(x)=w1412:dbl)
                    n1182 = Divide(x=w1412, y=w1411) -> (x/y=w1415:dbl)
                    n1183 = To Double Precision Float(number="Xpixels") -> (double precision float=w1410:dbl)
                    n1184 = Divide(x=w1410, y=w1415) -> (x/y=w1409:dbl)
                    n1185 = To Long Integer(number=w1409) -> (32bit integer=w1413:i32)
                    n1186 = local write "Xpixels"("Xpixels") -> ()
                    n1187 = local write "Ypixels"(w1413) -> ()
                  }
                  frame True {
                  }
                }
              }
            }
          }
          event "Ypixels": Value Change {
            n1188 = event-data() -> ()  [unwired: 1 in, 1 out]
            n1189 = local read "square pixels"() -> (w1422:bool)
            n1190 = case shown="True" w1422 {
              frame False {
                n1191 = local read "square matrix"() -> (w1423:bool)
                n1192 = case shown="True" w1423 {
                  frame False {
                  }
                  frame True {
                    n1193 = local read "Ypixels"() -> (w1424:i32)
                    n1194 = local write "Ypixels"(w1424) -> ()
                    n1195 = local write "Xpixels"(w1424) -> ()
                  }
                }
              }
              frame True {
                n1196 = local read "square matrix"() -> (w1425:bool)
                n1197 = case shown="False" w1425 {
                  frame False {
                    n1198 = local read "Vy-min"() -> (w1434:dbl)
                    n1199 = local read "Vx-max"() -> (w1438:dbl)
                    n1200 = local read "Vx-min"() -> (w1437:dbl)
                    n1201 = local read "Vy-max"() -> (w1433:dbl)
                    n1202 = Subtract(x=w1433, y=w1434) -> (x-y=w1435:dbl)
                    n1203 = Subtract(x=w1438, y=w1437) -> (x-y=w1436:dbl)
                    n1204 = Absolute Value(x=w1435) -> (abs(x)=w1429:dbl)
                    n1205 = Absolute Value(x=w1436) -> (abs(x)=w1430:dbl)
                    n1206 = Divide(x=w1430, y=w1429) -> (x/y=w1432:dbl)
                    n1207 = To Double Precision Float(number="Ypixels") -> (double precision float=w1427:dbl)
                    n1208 = Multiply(x=w1427, y=w1432) -> (x*y=w1426:dbl)
                    n1209 = To Long Integer(number=w1426) -> (32bit integer=w1431:i32)
                    n1210 = local write "Xpixels"(w1431) -> ()
                    n1211 = local write "Ypixels"("Ypixels") -> ()
                  }
                  frame True {
                  }
                }
              }
            }
          }
          event "Drawing Mode": Value Change {
            n1212 = event-data() -> ()  [unwired: 1 in, 6 out]
            n1213 = local write "Rotate"(FALSE) -> ()
          }
          event "reset angle": Value Change {
            n1214 = event-data() -> ()  [unwired: 1 in, 1 out]
          }
          event "no draw": Value Change {
            w1442 = FALSE
            n1215 = event-data() -> ()  [unwired: 1 in, 1 out]
            n1216 = property on="Rotate" class="Bool (strict)"("Value"=w1442) -> ()  [unwired: 2 in, 2 out]
            n1217 = property on="no draw" class="Bool (strict)"("DisabledEnum"=T2."Disabled" ("Disabled")) -> ()  [unwired: 2 in, 2 out]
            n1218 = property on="OK Button" class="Bool (strict)"("DisabledEnum"=T2."Enabled" ("Disabled")) -> ()  [unwired: 2 in, 2 out]
            n1219 = local write "no draw"(FALSE) -> ()
            n1220 = property on="no draw" class="Bool (strict)"("Visible"=w1442) -> ()  [unwired: 2 in, 2 out]
          }
          event "imageselect": Value Change {
            n1221 = event-data() -> ()  [unwired: 1 in, 6 out]
            n1222 = local read "imageselect"() -> (w1448:u16)
            n1223 = call "dattoimage.vi"("image2list"=w1448, "Current Average"=sgl 1.0, "image1list"=w1448) -> ("image 1 array out"=w1450:sgl[][])  [unwired: 1 out]
            n1224 = Transpose 2D Array(2D array=w1450) -> (transposed array=w1447:sgl[][])
            n1225 = local write "Image"(w1447) -> ()
          }
          event "OK Button": Value Change {
            n1226 = event-data() -> ()  [unwired: 1 in, 1 out]
            n1227 = case shown="True" "OK Button" {
              tunnel: [FALSE TRUE] -> w1451
              frame False {
              }
              frame True {
                n1228 = local read "Drawing Mode"() -> (w1454:u16)
                n1229 = case shown="1, Default" w1454 {
                  frame 0 {
                    n1230 = local read "Angle"() -> (w1458:dbl)
                    n1231 = local read "Drawing Mode"() -> (w1462:u16)
                    n1232 = local read "Scanning Mode"() -> (w1461:u16)
                    n1233 = local read "square matrix"() -> (w1476:bool)
                    n1234 = local read "square pixels"() -> (w1475:bool)
                    n1235 = local read "Vx-min"() -> (w1471:dbl)
                    n1236 = local read "Vx-max"() -> (w1470:dbl)
                    n1237 = local read "Vy-min"() -> (w1474:dbl)
                    n1238 = local read "Colormap"() -> (w1468:u16)
                    n1239 = local read "Ypixels"() -> (w1472:i32)
                    n1240 = local read "Vy-max"() -> (w1473:dbl)
                    n1241 = local read "Xpixels"() -> (w1469:i32)
                    n1242 = call "2pparameters.vi"("command"="get") -> ("params out"=w1464:T6)  [unwired: 1 in]
                    n1243 = Unbundle By Name(w1464) -> ("Angle Img"=w1459:dbl)
                    n1244 = Add(x=w1458, y=w1459) -> (x+y=w1463:dbl)
                    n1245 = Bundle By Name(cluster=w1464, "Scanning Mode"=w1461, "Drawing Mode"=w1462, "Xpixels Img"=w1469, "Vx-min Img"=w1471, "VX-max Img"=w1470, "Ypixels Img"=w1472, "Vy-min Img"=w1474, "Vy-max Img"=w1473, "Colormap"=w1468, "square pixels"=w1475, "square matrix"=w1476, "Angle Img"=w1463, "Angle draw"=0.0) -> (w1466:T6)
                    n1246 = call "2pparameters.vi"("Params in"=w1466, "command"="set") -> ()  [unwired: 1 out]
                  }
                  frame 1, Default {
                    n1247 = local read "Drawing Mode"() -> (w1480:u16)
                    n1248 = local read "Scanning Mode"() -> (w1479:u16)
                    n1249 = local read "square matrix"() -> (w1493:bool)
                    n1250 = local read "square pixels"() -> (w1492:bool)
                    n1251 = local read "Vx-min"() -> (w1488:dbl)
                    n1252 = local read "Vx-max"() -> (w1487:dbl)
                    n1253 = local read "Vy-min"() -> (w1491:dbl)
                    n1254 = local read "Colormap"() -> (w1485:u16)
                    n1255 = local read "Ypixels"() -> (w1489:i32)
                    n1256 = local read "Vy-max"() -> (w1490:dbl)
                    n1257 = local read "Xpixels"() -> (w1486:i32)
                    n1258 = local read "Angle"() -> (w1478:dbl)
                    n1259 = call "2pparameters.vi"("command"="get") -> ("params out"=w1481:T6)  [unwired: 1 in]
                    n1260 = Unbundle By Name(w1481) -> ("Angle Img"=w1477:dbl)
                    n1261 = Bundle By Name(cluster=w1481, "Scanning Mode"=w1479, "Drawing Mode"=w1480, "Xpixels"=w1486, "Vxminref"=w1488, "Vxmaxref"=w1487, "Ypixels"=w1489, "Vyminref"=w1491, "Vymaxref"=w1490, "Colormap"=w1485, "square pixels"=w1492, "square matrix"=w1493, "Angle Img"=w1477, "Angle draw"=w1478) -> (w1483:T6)
                    n1262 = call "2pparameters.vi"("Params in"=w1483, "command"="set") -> ()  [unwired: 1 out]
                  }
                }
                n1263 = call "ROI-databuffer.vi"("array in"="Array", "command"=enum16{"get", "set", "clear", "append"}."set") -> ()  [unwired: 3 in, 1 out]
              }
            }
          }
          event "Cancel Button": Value Change {
            n1264 = event-data() -> ()  [unwired: 1 in, 1 out]
            n1265 = case shown="True" "Cancel Button" {
              tunnel: [FALSE TRUE] -> w1494
              frame False {
              }
              frame True {
                n1266 = call "2pparameters.vi"("command"="get") -> ("params out"=w1500:T6)  [unwired: 1 in]
                n1267 = call "ROI-databuffer.vi"("command"=enum16{"get", "set", "clear", "append"}."get") -> ("array out"=w1499:cluster{"x":sgl, "y":sgl}[])  [unwired: 4 in]
                n1268 = call "2pparameters.vi"("Params in"=w1500, "command"="set") -> ()  [unwired: 1 out]
                n1269 = call "ROI-databuffer.vi"("array in"=w1499, "command"=enum16{"get", "set", "clear", "append"}."set") -> ()  [unwired: 3 in, 1 out]
              }
            }
          }
        }
        n1270 = Equal To 0?(x=w79) -> (x = 0?=w78:cluster{"Horizontal":bool, "Vertical":bool})
        n1271 = Unbundle(w78) -> ("Horizontal"=w77:bool, "Vertical"=w76:bool)
        n1272 = Equal To 0?(x=w86) -> (x = 0?=w90:cluster{"Horizontal":bool, "Vertical":bool})
        n1273 = Equal To 0?(x=w83) -> (x = 0?=w84:bool)
        n1274 = Unbundle(w90) -> ("Horizontal"=w89:bool, "Vertical"=w88:bool)
        n1275 = And(x=w77, y=w76) -> (x .and. y?=w81:bool)
        n1276 = And(x=w89, y=w88) -> (x .and. y?=w87:bool)
        n1277 = Select(t=w72, s=w84, f=w83) -> (s? t:f=w82:dbl)
        n1278 = Select(t=w63, s=w81, f=w79) -> (s? t:f=w80:T1)
        n1279 = Select(t=w64, s=w87, f=w86) -> (s? t:f=w85:T1)
      }
    }
  }
